vi "FrontPanel-4.50-backup.vi"() -> ()   [LabVIEW 2013]
doc: "This VI controls the blindpanel type GHS-2T-1T-700 for a CryoFree DR. Automatization control is embedded in the blindpanel. Keys can be manipulated from within this VI."
uses:
  Leiden to DSC/FP to DSC/Typedefs/FP-cluster.ctl
  1. Sources/Lib/Lib.llb/ErrCodeStatusLkup.vi
  1. Sources/Lib/Lib.llb/Pfeiffer Vacuum.lvlib
  1. Sources/Lib/Lib.llb/MView.lvlib
  1. Sources/Lib/Lib.llb/Busy PopUp.lvlib
panel:
  out "VIRef":T1 {"Array DataType" format="%.0x"; "WaveForm Type" format="%.0x"; "RefNum Type" format="%.0x"; "DataType" format="%.0x"}
  out "ControlNames":string[](array[string])
  in  "Toolbar":enum32{"Page 1", "Page 2"}(tab)
  in  "Load config":bool
  in  "Save config":bool
  in  "Start":bool
  in  "Stop":bool
  out "V":string
  out "PT2 Data":dbl[](array[numeric])
  in  "Restart PT on Error?":bool
  in  "Attempts":u16=6
  in  "Time delay":u16=60 format="%.0f s"
  out "Error Log":string[][](table)
  in  "Error panel":enum32{"Page 1"}(tab)
  out "PT2 error":errorcluster
  out "MG error":errorcluster
  out "PT1 error":errorcluster
  out "FP error":errorcluster
  out "PT1 Data":dbl[](array[numeric])
  in  "Main Panel":enum32{"Page 1", "Page 2"}(tab)
  out "PC":sgl
  out "P1":sgl format="%.1f"
  out "P2":sgl format="%.1f"
  out "P3":sgl format="%.1f"
  out "P4":sgl format="%.1f"
  out "P5":sgl format="%.1f"
  out "P6":sgl format="%.1f"
  out "P7":sgl format="%.1f"
  out "Flow":sgl format="%#_4f"
  out "P5 alarm":bool
  out "Pstill (P8)":dbl format="%.1e"
  in  "Main Panel":T2(tab)
  out "String 2":string
  out "String 4":string
  out "String":string
  out "String 3":string
  out "Mode":u16(ring) items=["AUTO MODE OFF", "START", "CONDENSING 3He", "CONDENSING 4He", "NORMAL CIRCULATION", "RECOVERY OF THE MIXTURE", "RECOVERY: BLOCKAGE OR OVERPRESSURE"]
  out "FLOW":sgl format="%#_3f"
  out "P5":sgl
  out "P4":sgl
  out "P3":sgl
  out "P1":sgl
  out "P2":sgl
  out "3He":sgl(slide) min=0 max=2 scale=0.0..2000.0 scale format="%.2f"
  out "4He":sgl(slide) min=0 max=2 scale=0.0..2000.0 scale format="%.2f"
  out "Panel ID":string
  in  "FP type":enum32{"OLD", "NEW"}(tab)
  in  "Buttons":T3
  out "LEDs":T4
  in  "Buttons 2":T3
  out "LEDs 2":T5
  out "PC":sgl
  in  "PT Start 2":bool
  in  "PT_stop 2":bool
  in  "PT2 Plots Select":T6
  out "PT2 Status":cluster{"Time":dbl[], "Value":dbl[]}[](graph)
  in  "PT_ResetValues 2":bool
  out "PT Error Code 2":i32 caption="PT Error Code"
  out "PT Error 2":string="NO ERROR" caption="PT Error"
  out "P High":cluster{dbl, dbl, dbl, dbl}(slide) scale=150.0..450.0
  out "P Low":cluster{dbl, dbl, dbl, dbl}(slide) scale=0.0..300.0
  out "P_avg 2":cluster{"Low":dbl, "High":dbl} caption="Average pressure"
  out "Helium":cluster{dbl, dbl, dbl, dbl}(slide) scale=0.0..95.0
  out "Water In":cluster{dbl, dbl, dbl, dbl}(slide) scale=0.0..35.0
  out "Water Out":cluster{dbl, dbl, dbl, dbl}(slide) scale=0.0..60.0
  out "PT Status":u16(ring) items=["Compressor OFF", "Compressor ON", ""]
  out "Motor":cluster{dbl, dbl}(slide) scale=0.0..30.0
  out "Oil":cluster{dbl, dbl, dbl, dbl}(slide) scale=0.0..60.0
  in  "PT1 Plots Select":T6
  out "PT1 Status 2":cluster{"Time":dbl[], "Value":dbl[]}[](graph)
  out "P Low":cluster{dbl, dbl, dbl, dbl}(slide) scale=0.0..300.0
  out "P High":cluster{dbl, dbl, dbl, dbl}(slide) scale=150.0..450.0
  out "P_avg":cluster{"Low":dbl, "High":dbl} caption="Average pressure"
  out "Motor":cluster{dbl, dbl}(slide) scale=0.0..30.0
  out "Oil":cluster{dbl, dbl, dbl, dbl}(slide) scale=0.0..60.0
  out "Helium":cluster{dbl, dbl, dbl, dbl}(slide) scale=0.0..95.0
  out "Water Out":cluster{dbl, dbl, dbl, dbl}(slide) scale=0.0..60.0
  out "Water In":cluster{dbl, dbl, dbl, dbl}(slide) scale=0.0..35.0
  out "PT Error Code":i32
  out "PT Error":string="NO ERROR"
  in  "PT_ResetValues":bool
  in  "PT Start":bool
  in  "PT_stop":bool
  out "PT Status":u16(ring) items=["Compressor OFF", "Compressor ON", ""]
  in  "MG Plots Select":T6
  in  "FP Plots Select":T6
  out "MaxiGauge":cluster{"Time":dbl[], "Value":dbl[]}[](graph)
  out "Front Panel":cluster{"Time":dbl[], "Value":dbl[]}[](graph)
  in  "Boolean 2":bool
  out "PT2 port":u16
  out "PT1 port":u16
  out "MG port":refnum<visa-resource-name>="COM4" caption="Port number"
  out "FP port":refnum<visa-resource-name>="COM3" caption="Port number"
  out "ForceSave":bool
  in  "Button":u8
  out "SetControl":T7
  in  "S2":enum32{"Page 1"}(tab)
  in  "Reset Error 2":bool
  in  "S1":enum32{"Page 1"}(tab)
  in  "Reset Error":bool
  out "Cur Path":path
  in  "Side Panel":enum32{"Main", "Settings", "Advanced"}(tab)=enum."Settings"
  out "Maxigauge ID":string caption="ID"
  out "Panel response":string
  out "Sensors Status":T8={"String 8"="OK", "String 9"="OK", "String 10"="OK", "String 11"="OK", "String 12"="OK", "String 13"="OK"}
  in  "ADC scaling":T9={"P1"=2500.0, "P2"=2500.0, "P3"=2500.0, "P4"=2500.0, "P5"=2500.0, "P6"=2500.0, "P7"=2500.0, "Flow meter"=682.0, "PC"=10000.0} caption="Front panel ADC scaling factors" {"Flow meter" format="%#.4f"}
  in  "REC Settings":T10={"P6 low"=20, "P6 high"=1000, "P7 low"=20}
  in  "NCP5B Settings":cluster{"P6 low":u16}={"P6 low"=20}
  in  "NCP5 Settings":T10={"P6 low"=20, "P6 high"=1000, "P7 low"=20}
  in  "S1&2 Settings":cluster{"Enum":enum16{"OFF", "ON"}}
  in  "P5 Settings":cluster{"P6 low":u16, "P6 high":u16}={"P6 low"=20, "P6 high"=1000}
  out "REC limits":T11={"P5 warn"=20, "P5 rec"=20, "P5 res"=20}
  out "NCP5B limits":cluster{"P5 NC4":u16}={"P5 NC4"=20}
  out "NCP5 limits":T12={"P5 NC1"=20, "P5 NC2"=20, "P5 NC3"=20}
  out "S1&2 limits":cluster{"S1&S2":enum16{"OFF", "ON"}}
  out "P5 limits":cluster{"P5 C1":u16, "P5 C2":u16}={"P5 C1"=20, "P5 C2"=20}
  in  "P6&7 Settings":T13={"P6 low"=20, "P6 high"=1600, "P7 low"=20, "P7 high"=1610}
  out "P6&7 limits":T13={"P6 low"=20, "P6 high"=20, "P7 low"=20, "P7 high"=20}
  in  "SET VALUES":bool
  out "MG pressures":T14 {"Channel 1" format="%-7.2e mbar"; "Channel 1" format="%-7.2e mbar"; "Channel 1" format="%-7.2e mbar"; "Channel 1" format="%-7.2e mbar"; "Channel 1" format="%-7.2e mbar"; "Channel 1" format="%-7.2e mbar"}
  out "Cluster":T15={"String 2"="\"\"", "String 3"="", "String 4"="", "String 5"="", "String 6"="", "String 7"=""}
  in  "Log Options":T16={"Plot data "=TRUE, "Every1"=1.0, "Save to log"=TRUE, "Every  2"=1.0, "AVS_Path 2"=path "C:/LC Data/Data", "AVS_FName"="logFP", "Filename suffix"="_%Y-%m-%d-%H-%M-%S", "NewFevery"=7, "Time Units"=enum."Days", "Date Format"="%Y-%m-%d %H:%M:%S", "Averages"=4} caption="Data Logging \nOptions" {"Every  2" format="%#_g min"; "Every1" format="%#_g min"}
  in  "Configuration":T17={"FP port number"="COM3", "MG port number"="COM4", "PT1 Enabled?"=FALSE, "MG  channel P8"=65535, "Stop auto recovery if still is empty"=FALSE, "PT1 port number"="COM2", "MG Enabled?"=TRUE, "PT1 Address"=16, "S1 Enabled?"=FALSE, "S1 port"="COM2", "S2 Enabled?"=FALSE, "S2 port"="COM2", "Device address S1"=1, "Device address S2"=2, "PT1 Bauds"=115200, "PT2 Enabled?"=FALSE, "PT2 port number"="COM2", "PT2 Address"=16, "PT2 Bauds"=115200, "FP baud rate"=9600} {"PT2 Address" min=16 max=126 step=1; "MG  channel P8" items=["Channel 1", "Channel 2", "Channel 3", "Channel 4", "Channel 5", "Channel 6"]; "PT1 Address" min=16 max=126 step=1}
  in  "Type":enum32{"Wet", "CF"}(radio)=enum."CF"
  in  "Panel Layout":enum32{"OLD", "NEW"}(ring)=enum."NEW"
  out "RAW ADC Values 2":dbl[](array[numeric]) caption="Converted ADC Values"
  in  "SendCMD":bool caption="Send"
  out "Response":string
  in  "Command":string
  out "SP reached? 2":bool
  in  "Cond1":bool
  in  "Delay Time":u32=30 caption="For a time delay of" format="%.0f min"
  in  "MG  channel":u16(ring)=65535 caption="MaxiGauge" items=["Channel 1", "Channel 2", "Channel 3", "Channel 4", "Channel 5", "Channel 6"]
  out "SP reached? 3":bool
  in  "P threshold":dbl=0.0005 caption="<" format="%#_2g mbar"
  in  "Cond2":bool
  out "SP reached?":bool
  out "Delay Timer":u32=10 caption="Timer" format="%<%M:%S>t"
  in  "EnableAutoCond":bool caption="Start"
  out "VI path":string
  out "RAW ADC Values":i32[](array[numeric])
  in  "Autoconf":bool caption="Autoconfigure"
  out "MG Data":dbl[](array[numeric]) format="%.3e"
  out "FP Data":sgl[](array[numeric]) format="%.2f"
  out "FP Status bits":u32[](array[numeric])
  out "Attempts Counter":u16
  # "Error log"
  # "Front panel status"
  # "MaxiGauge status"
  # "Pulse Tube 1 status"
  # "Pulse Tube 2 status"
  # "Leiden Cryogenics"
  # "to \nair"
  # "N.C."
  # "from\novc"
  # "from\nivc"
  # "from still"
  # "to 3He\nin-1"
  # "to 3He\nin-2"
  # "P8"
  # "AUX 1"
  # "BYPASS"
  # "MIXTURE\nCOMPRESSOR"
  # "M2"
  # "P6"
  # "M3"
  # "M1"
  # "AUX PORT-1"
  # "P7"
  # "TRAP"
  # "AUX TRAP"
  # "To \nAir"
  # "From\nIVC"
  # "From Still"
  # "To 3He\nin-1"
  # "To 3He\nin-2"
  # "To \nAir"
  # "N.C."
  # "from\novc"
  # "from\nivc"
  # "from still"
  # "to 3He\nin-1"
  # "to 3He\nin-2"
  # "Leiden Cryogenics"
  # "to \nair"
  # "N.C."
  # "from\novc"
  # "from\nivc"
  # "from still"
  # "to 3He\nin-1"
  # "to 3He\nin-2"
  # "P8"
  # "M2"
  # "P6"
  # "M3"
  # "TRAP"
  # "AUX TRAP"
  # "M1"
  # "AUX PORT-1"
  # "P7"
  # "AUX 1"
  # "To \nAir"
  # "From\nIVC"
  # "From Still"
  # "To 3He\nin-1"
  # "to 3He\nin-1"
  # "To 3He\nin-2"
  # "to \nair"
  # "N.C."
  # "from\novc"
  # "from\nivc"
  # "from still"
  # "to 3He\nin-2"
  # "Pulse Tube 1"
  # "Pulse Tube 2"
  # "Front Panel"
  # "MaxiGauge"
  # "Turbo2 (S2)"
  # "Turbo1 (S1)"
  # "MaxiGauge"
  # "#"
  # "NAME"
  # "PRESSURE"
  # "STATUS"
  # "1"
  # "2"
  # "3"
  # "4"
  # "5"
  # "6"
  # "Automatic mode pressure limits"
  # "Warning: These values influence the operation of the GHS in automatic mode. Please refer to the operation manual and consult with Leiden Cryogenics before changing them."
  # "NAME"
  # "FW"
  # "NEW"
  # "DESCRIPTION"
  # "Stop condensing 4He"
  # "Stop recovering 4He"
  # "Stop condensing 3He"
  # "Stop recovering 3He"
  # "Condensing->open 12"
  # "Condensing->close 9/12"
  # "Condensing->run S1&S2"
  # "NC->open second line"
  # "NC->start MC"
  # "NC->open aux. trap"
  # "NC->stop MC, close 7"
  # "All->P5 alarm"
  # "All->switch to recovery"
  # "All->reset"
  # "Front panel ADC scaling factors"
  # "Data Logging and Plotting"
  # "Front Panel"
  # "MaxiGauge"
  # "Pulse Tube 1"
  # "Pulse Tube 2"
  # "Turbo 1 (S1) (Pfeiffer HiPACE only)"
  # "Turbo2 (S2) (Pfeiffer HiPACE only)"
  # "Automatic condensing"
  # "Start condensing when"
  # "and wait"
  # "Send command to Front Panel"
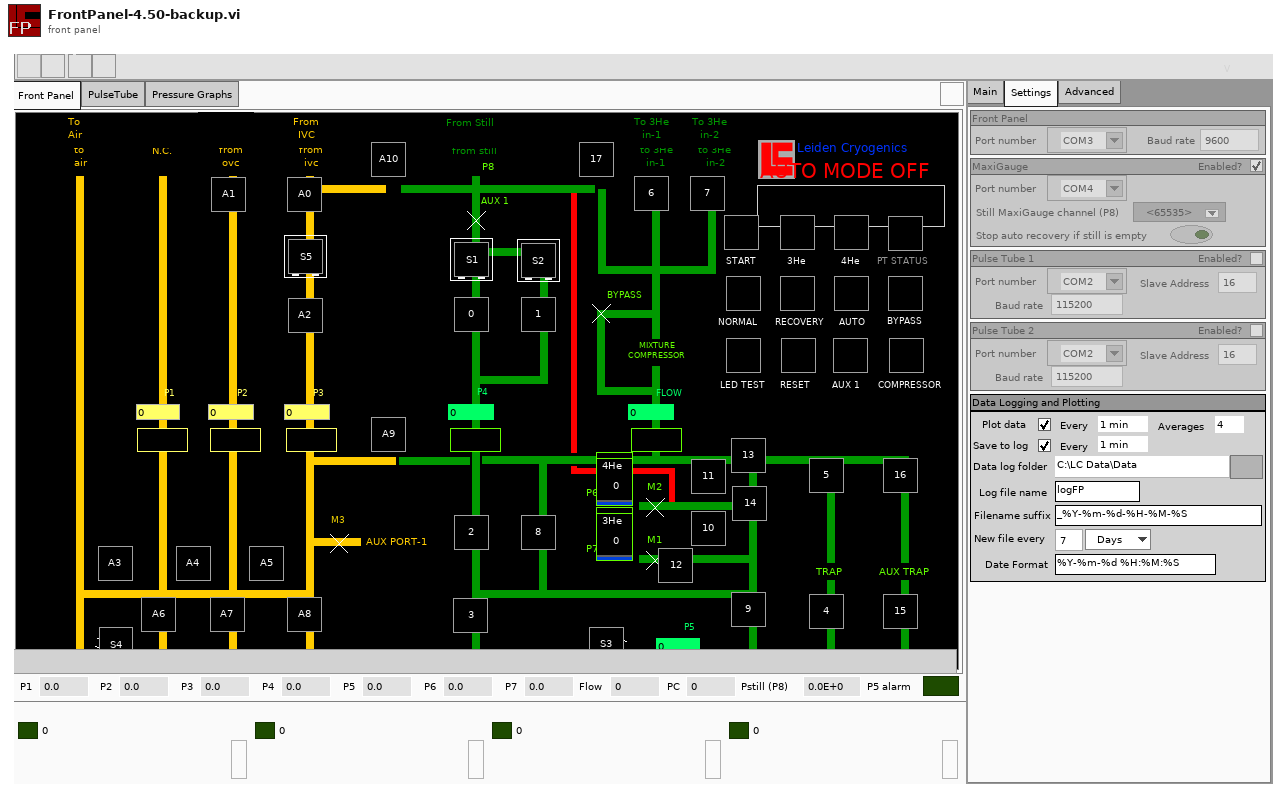
[diagram p1: front panel]
types:
  T1 = cluster{"Control Ref ID":refnum<vi>[], "Full Name":string[], "ClassID":enum16{"<Null>", "1", "2", "Generic", "Decoration", "Text", "Control", "ColorBox", "Boolean", "RefNum", "Variant", "Path", "ListBox", "Table", "Array", "Picture", "ActiveXContainer", "Numeric", "Digital", "NamedNumeric", "ColorRamp", "Slide", "GraphOrChart", "WaveformChart", "WaveformGraph", "IntensityChart", "IntensityGraph", "String", "IOName", "ComboBox", "Cluster", "Panel", "Knob", "NumWithScale", "Ring", "Enum", "GObject", "Plot", "Cursor", "NumericText", "Scale", "ColorScale", "GraphScale", "ColorGraphScale", "TypedRefNum", "OldKnobScale", "MCListbox", "MeasureData", "BVTag", "DAQName", "VISAName", "IVIName", "SlideScale", "TabControl", "Page", "TabArrayTabControl", "ConPane", "57", "58", "59", "60", "61", "62", "63", "64", "SubPanel", "TreeControl", "67", "68", "69", "70", "71", "72", "73", "74", "75", "SplitterBar"}[], "Short Name":string[], "DataType":enum8{"<Null>", "I8", "I16", "I32", "I64", "U8", "U16", "U32", "U64", "SGL", "DBL", "EXT", "CSG", "CDB", "CXT", "0x0F", "0x10", "0x11", "0x12", "0x13", "0x14", "Enum U8", "Enum U16", "Enum U32", "Enum U64", "SGL PQ", "DBL PQ", "EXT PQ", "CSG PQ", "CDB PQ", "CXT PQ", "0x1F", "0x20", "Boolean", "0x22", "0x23", "0x24", "0x25", "0x26", "0x27", "0x28", "0x29", "0x2A", "0x2B", "0x2C", "0x2D", "0x2E", "0x2F", "String", "0x31", "Path", "Pict", "0x34", "0x35", "0x36", "DAQ", "0x38", "0x39", "0x3A", "0x3B", "0x3C", "0x3D", "0x3E", "0x3F", "Array", "0x41", "0x42", "0x43", "0x44", "0x45", "0x46", "0x47", "0x48", "0x49", "0x4A", "0x4B", "0x4C", "0x4D", "0x4E", "0x4F", "Cluster", "0x51", "0x52", "Variant", "Waveform", "0x55", "0x56", "0x57", "0x58", "0x59", "0x5A", "0x5B", "0x5C", "0x5D", "0x5E", "0x5F", "0x60", "0x61", "0x62", "0x63", "0x64", "0x65", "0x66", "0x67", "0x68", "0x69", "0x6A", "0x6B", "0x6C", "0x6D", "0x6E", "0x6F", "Refnum"}[], "RefNum Type":enum8{"Generic", "Datalog File Refnum", "Byte Stream File Refnum", "Device Refnum", "Occurence Refnum", "TCP Connection Refnum", "VISA Refnum (Obsolete)", "Automation Renum", "VI Server Refnum", "Menu Refnum", "IVI Refnum (Obsolete)", "IMAQ Session", "0x0C", "Datasocket Refnum", "VISA Resource", "IVI Logical Name", "UDP Connection Refnum", "Notifier Refnum", "Queue Refnum", "IrDA Refnum", "Hardware Plugin Refnum", "Hardware Plugin Tag Refnum", "DAQmx Refnum", "Event Registration Refnum", ".NET Refnum", "User Event Refnum", "0x1A", "Event Callback", "0x1C", "0x1D", "Only Used Internal to LabVIEW", "Bluetooth", "Data Value References", "RT FIFO", "TDM Streaming"}[], "WaveForm Type":enum8{"<Not a Waveform Type>", "0x01", "Analog 16-bit signed", "Analog Double-Precision", "0x04", "Analog Single Precision", "Timestamp", "Digital Data", "Digital Waveform", "Dynamic Data", "Analog Extended-Precision", "Analog 8-bit unsigned", "Analog 16-bit unsigned", "Analog 32-bit unsigned", "Analog 8-bit signed", "Analog 32-bit signed", "Analog Complex Single-Precision", "Analog Complex Double-Precision", "Analog Complex Extended Precision", "Analog 64-bit signed", "Analog 64-bit unsigned"}[], "Parent":i32[], "Array DataType":enum8{"<Null>", "I8", "I16", "I32", "I64", "U8", "U16", "U32", "U64", "SGL", "DBL", "EXT", "CSG", "CDB", "CXT", "0x0F", "0x10", "0x11", "0x12", "0x13", "0x14", "Enum U8", "Enum U16", "Enum U32", "Enum U64", "SGL PQ", "DBL PQ", "EXT PQ", "CSG PQ", "CDB PQ", "CXT PQ", "0x1F", "0x20", "Boolean", "0x22", "0x23", "0x24", "0x25", "0x26", "0x27", "0x28", "0x29", "0x2A", "0x2B", "0x2C", "0x2D", "0x2E", "0x2F", "String", "0x31", "Path", "Pict", "0x34", "0x35", "0x36", "DAQ", "0x38", "0x39", "0x3A", "0x3B", "0x3C", "0x3D", "0x3E", "0x3F", "Array", "0x41", "0x42", "0x43", "0x44", "0x45", "0x46", "0x47", "0x48", "0x49", "0x4A", "0x4B", "0x4C", "0x4D", "0x4E", "0x4F", "Cluster", "0x51", "0x52", "Variant", "Waveform", "0x55", "0x56", "0x57", "0x58", "0x59", "0x5A", "0x5B", "0x5C", "0x5D", "0x5E", "0x5F", "0x60", "0x61", "0x62", "0x63", "0x64", "0x65", "0x66", "0x67", "0x68", "0x69", "0x6A", "0x6B", "0x6C", "0x6D", "0x6E", "0x6F", "Refnum"}[], "Owning VI":refnum<vi>[], "Active?":bool[]}
  T2 = enum32{"Front Panel", "PulseTube", "Pressure Graphs"}
  T3 = cluster{"baux2":bool, "bBypass":bool, "b15":bool, "b16":bool, "NC 0":bool, "baux1":bool, "b4":bool, "NC 1":bool, "b5":bool, "breset":bool, "NC 2":bool, "b9":bool, "b14":bool, "NC 3":bool, "b13":bool, "bledtest":bool, "NC 4":bool, "b12":bool, "b10":bool, "NC 5":bool, "b11":bool, "bA0":bool, "NC 9":bool, "b7":bool, "bS3":bool, "NC 12":bool, "b6":bool, "b17":bool, "NC 13":bool, "b8":bool, "b1":bool, "NC 14":bool, "bS2":bool, "b3":bool, "NC 15":bool, "b2":bool, "b0":bool, "NC 16":bool, "bS1":bool, "bA9":bool, "NC 17":bool, "bA8":bool, "bA2":bool, "NC 6":bool, "bs5":bool, "bA10":bool, "NC 7":bool, "bstart":bool, "bA5":bool, "NC 8":bool, "bA7":bool, "bA1":bool, "NC 10":bool, "bauto":bool, "bA4":bool, "NC 11":bool, "bA6":bool, "bS4":bool, "NC 18":bool, "bA3":bool, "b3he":bool, "b4he":bool, "bnorm":bool, "brecov":bool}
  T4 = cluster{"COMPR/AUX 2":bool, "BYPASS":bool, "15":bool, "16":bool, "NC 0":bool, "AUX 1":bool, "4":bool, "NC 1":bool, "5":bool, "RESET":bool, "NC 2":bool, "9":bool, "14":bool, "NC 3":bool, "13":bool, "LED TEST":bool, "NC 4":bool, "12":bool, "10":bool, "NC 5":bool, "11":bool, "A0":bool, "NC 12":bool, "7":bool, "S3":bool, "NC 13":bool, "6":bool, "17":bool, "NC 14":bool, "8":bool, "1":bool, "NC 15":bool, "S2":bool, "3":bool, "NC 16":bool, "2":bool, "0":bool, "NC 17":bool, "S1":bool, "A9":bool, "NC 6":bool, "A8":bool, "A2":bool, "NC 7":bool, "S5":bool, "A10":bool, "NC 8":bool, "START":bool, "A5":bool, "NC 9":bool, "A7":bool, "A1":bool, "NC 10":bool, "AUTO":bool, "A4":bool, "NC 11":bool, "A6":bool, "S4":bool, "NC 18":bool, "A3":bool, "3He":bool, "4He":bool, "NORMAL":bool, "RECOVERY":bool, "PT STATUS":bool}
  T5 = cluster{"COMPR/AUX 2":bool, "BYPASS":bool, "15":bool, "16":bool, "AUX 1":bool, "AUX 1":bool, "4":bool, "AUX 2":bool, "5":bool, "RESET":bool, "AUX 3":bool, "9":bool, "14":bool, "NC 3":bool, "13":bool, "LED TEST":bool, "NC 4":bool, "12":bool, "10":bool, "NC 5":bool, "11":bool, "A0":bool, "NC 12":bool, "7":bool, "S3":bool, "NC 13":bool, "6":bool, "17":bool, "NC 14":bool, "8":bool, "1":bool, "NC 15":bool, "S2":bool, "3":bool, "NC 16":bool, "2":bool, "0":bool, "NC 17":bool, "S1":bool, "A9":bool, "NC 6":bool, "A8":bool, "A2":bool, "NC 7":bool, "S5":bool, "A10":bool, "NC 8":bool, "START":bool, "A5":bool, "NC 9":bool, "A7":bool, "A1":bool, "NC 10":bool, "AUTO":bool, "A4":bool, "NC 11":bool, "A6":bool, "S4":bool, "NC 18":bool, "A3":bool, "3He":bool, "4He":bool, "NORMAL":bool, "RECOVERY":bool, "PT STATUS":bool}
  T6 = cluster{"Boolean":bool, "Boolean 2":bool, "Boolean 3":bool, "Boolean 4":bool, "Boolean 5":bool, "Boolean 6":bool, "Boolean 7":bool, "Boolean 8":bool}
  T7 = cluster{"Name":string, "Scalar":string, "Array":string[][]}
  T8 = cluster{"String 8":string, "String 9":string, "String 10":string, "String 11":string, "String 12":string, "String 13":string}
  T9 = cluster{"P1":dbl, "P2":dbl, "P3":dbl, "P4":dbl, "P5":dbl, "P6":dbl, "P7":dbl, "Flow meter":dbl, "PC":dbl}
  T10 = cluster{"P6 low":u16, "P6 high":u16, "P7 low":u16}
  T11 = cluster{"P5 warn":u16, "P5 rec":u16, "P5 res":u16}
  T12 = cluster{"P5 NC1":u16, "P5 NC2":u16, "P5 NC3":u16}
  T13 = cluster{"P6 low":u16, "P6 high":u16, "P7 low":u16, "P7 high":u16}
  T14 = cluster{"Channel 1":dbl, "Channel 1":dbl, "Channel 1":dbl, "Channel 1":dbl, "Channel 1":dbl, "Channel 1":dbl}
  T15 = cluster{"String 2":string, "String 3":string, "String 4":string, "String 5":string, "String 6":string, "String 7":string}
  T16 = cluster{"Plot data ":bool, "Every1":dbl, "Save to log":bool, "Every  2":dbl, "AVS_Path 2":path, "AVS_FName":string, "Filename suffix":string, "NewFevery":u32, "Time Units":enum16{"Minutes", "Hours", "Days"}, "Date Format":string, "Averages":i32}
  T17 = cluster{"FP port number":refnum<visa-resource-name>, "MG port number":refnum<visa-resource-name>, "PT1 Enabled?":bool, "MG  channel P8":u16, "Stop auto recovery if still is empty":bool, "PT1 port number":refnum<visa-resource-name>, "MG Enabled?":bool, "PT1 Address":u8, "S1 Enabled?":bool, "S1 port":refnum<visa-resource-name>, "S2 Enabled?":bool, "S2 port":refnum<visa-resource-name>, "Device address S1":u8, "Device address S2":u8, "PT1 Bauds":u32, "PT2 Enabled?":bool, "PT2 port number":refnum<visa-resource-name>, "PT2 Address":u8, "PT2 Bauds":u32, "FP baud rate":u32}
  T18 = cluster{"error":bool, "code":i32, "source":string}
  T19 = cluster{"Dict. Var":u16, "Description":string, "Values":i32[]}[]
  T20 = cluster{"[3]":dbl, "[3]":dbl, "[3]":dbl, "Values[3] 2":dbl}
  T21 = cluster{"[1]":dbl, "[1]":dbl, "[1]":dbl, "Values[1] 2":dbl}
  T22 = cluster{"Values[0]":dbl, "Values[0]":dbl, "Values[0]":dbl, "Values[0] 2":dbl}
  T23 = cluster{"error":bool, "code":i32, "error source":string}
  T24 = cluster{"sensor status info[0]":string, "sensor status info[1]":string, "sensor status info[2]":string, "sensor status info[3]":string, "sensor status info[4]":string, "sensor status info[5]":string}
  T25 = cluster{"Filterred[0]":dbl, "Filterred[1]":dbl, "Filterred[2]":dbl, "Filterred[3]":dbl, "Filterred[4]":dbl, "Filterred[5]":dbl}
  T26 = typedef "FP-cluster.ctl" = cluster{"FP Data":sgl[], "MG Data":dbl[], "PT Data":dbl[], "FP Status Bits":u32[], "Mode":u16}
  T27 = cluster{"FP Data[0]":sgl, "FP Data[1]":sgl, "FP Data[2]":sgl, "FP Data[3]":sgl, "FP Data[4]":sgl, "FP Data[5]":sgl, "FP Data[6]":sgl, "FP Data[7]":sgl, "FP Data[8]":sgl}
  T28 = enum32{"Page Enabled", "Page Disabled", "Page Disabled & Grayed"}
  T29 = enum32{"invalid app kind", "Development System", "Run Time System", "Student Edition", "Embedded LabVIEW", "Evaluation", "Custom"}
  T30 = cluster{"array of 4 x 16 bit unsigned[0]":u16, "array of 4 x 16 bit unsigned[1]":u16, "array of 4 x 16 bit unsigned[2]":u16, "array of 4 x 16 bit unsigned[3]":u16}
  T31 = cluster{"array of 2 x 16 bit unsigned[0]":u16, "array of 2 x 16 bit unsigned[1]":u16}
  T32 = cluster{"array of 3 x 16 bit unsigned[0]":u16, "array of 3 x 16 bit unsigned[1]":u16, "array of 3 x 16 bit unsigned[2]":u16}
  T33 = cluster{"Array[0]":string, "Array[1]":string, "Array[2]":string, "Array[3]":string, "Array[4]":string, "Array[5]":string}
  T34 = typedef "LVRectTypeDef.ctl" = cluster{"Left":i16, "Top":i16, "Right":i16, "Bottom":i16}
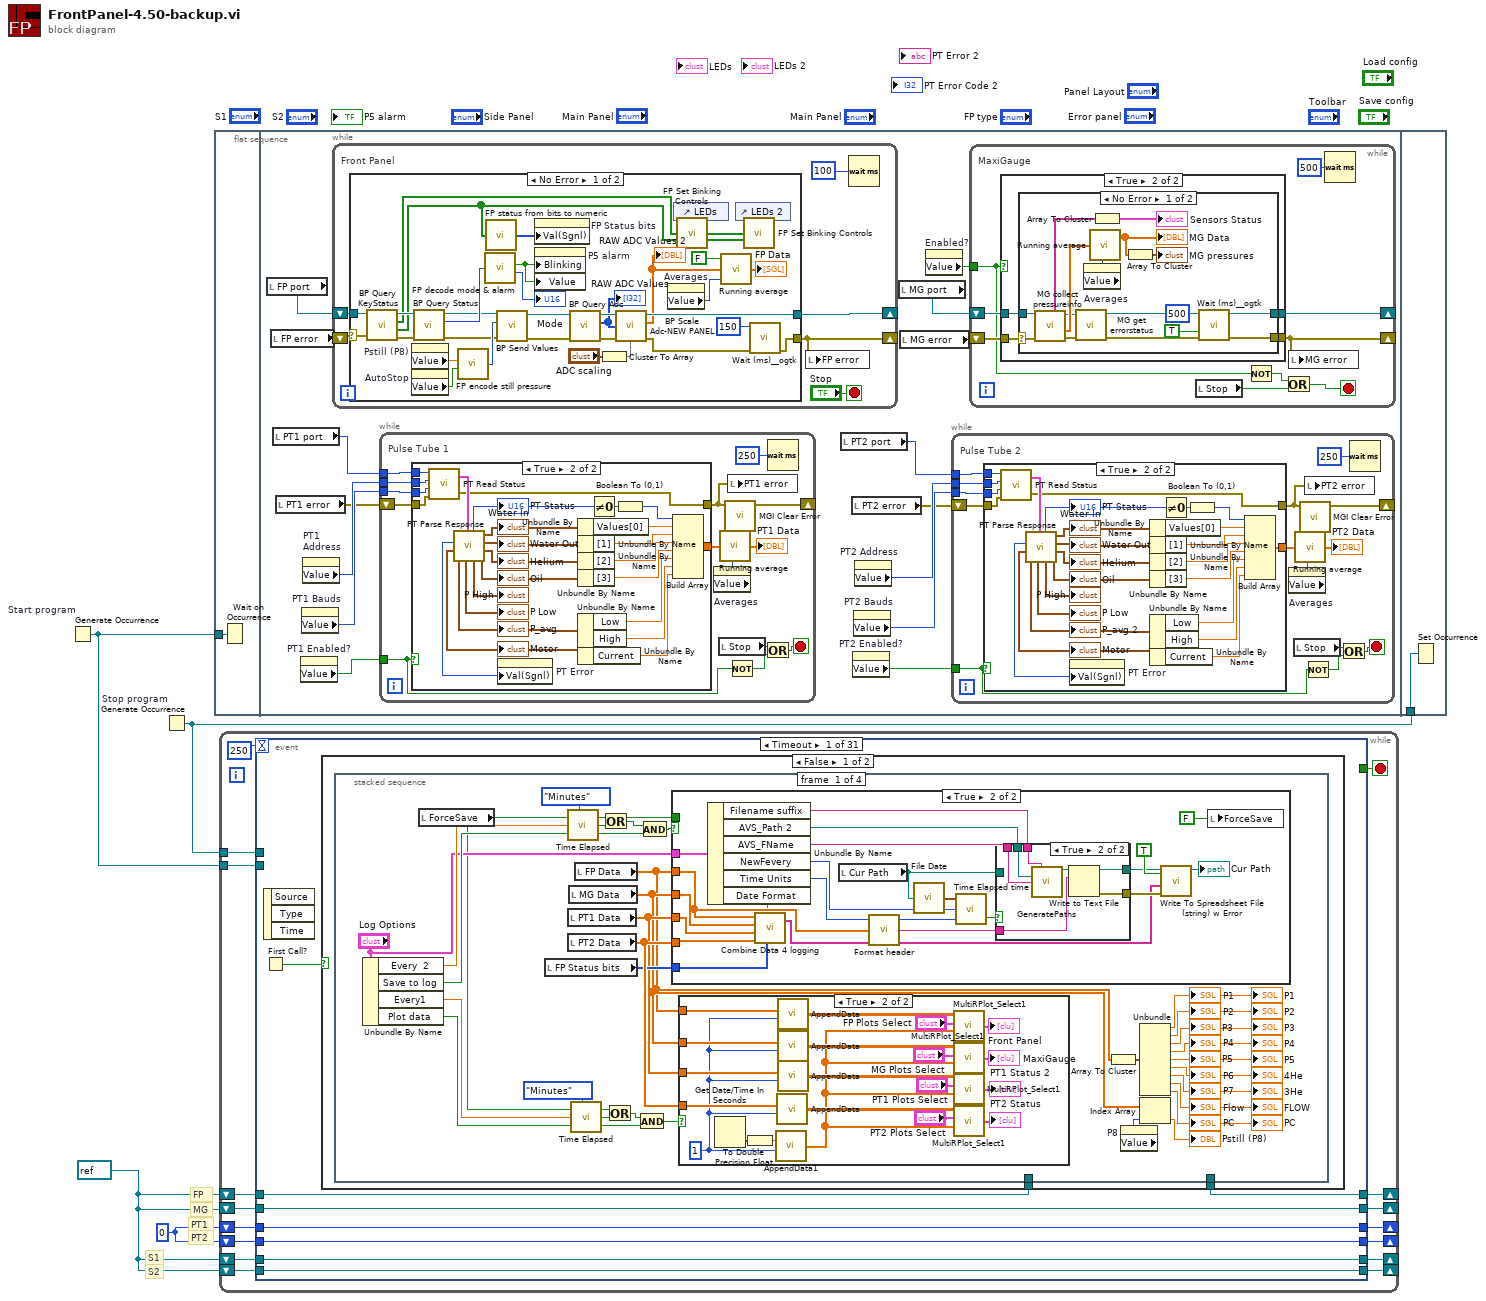
[diagram p0: block diagram]
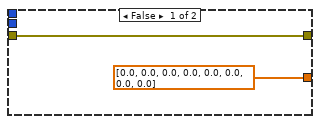
[diagram p2: hidden frame]
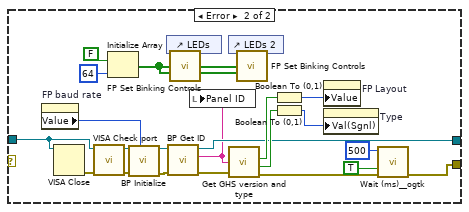
[diagram p3: hidden frame]
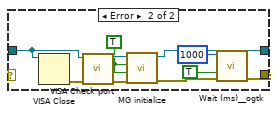
[diagram p5: hidden frame]
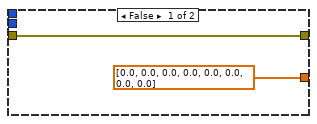
[diagram p6: hidden frame]
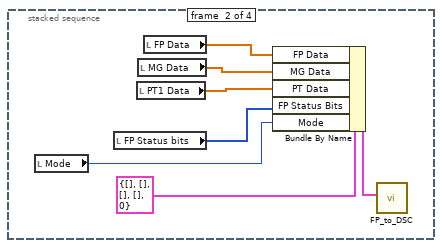
[diagram p10: hidden frame]
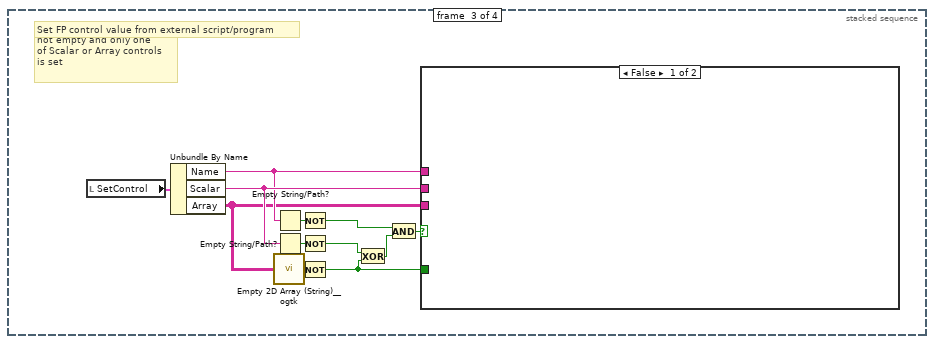
[diagram p11: hidden frame]
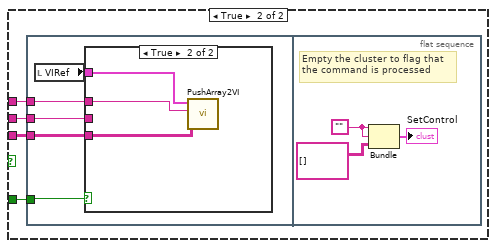
[diagram p12: hidden frame]
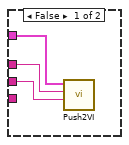
[diagram p13: hidden frame]
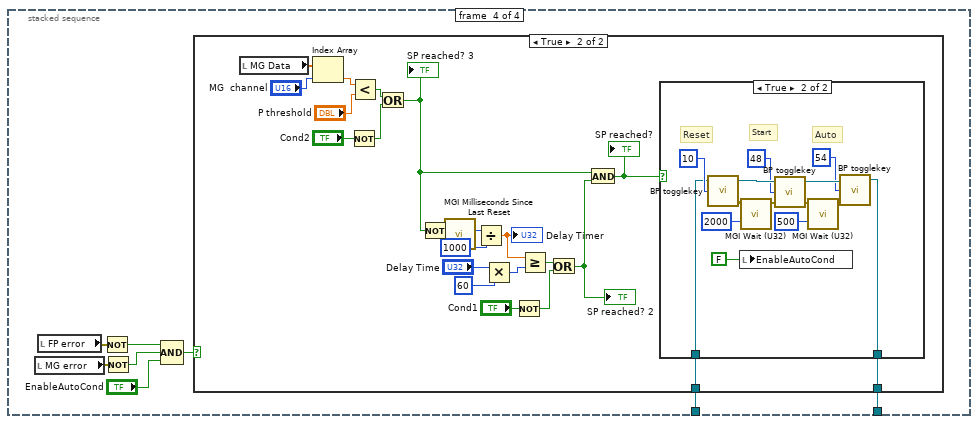
[diagram p14: hidden frame]
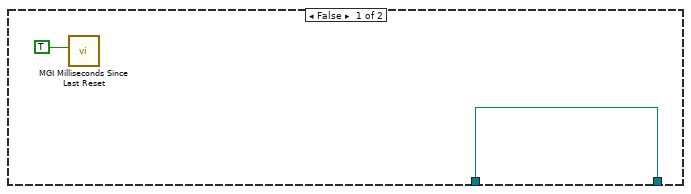
[diagram p15: hidden frame]
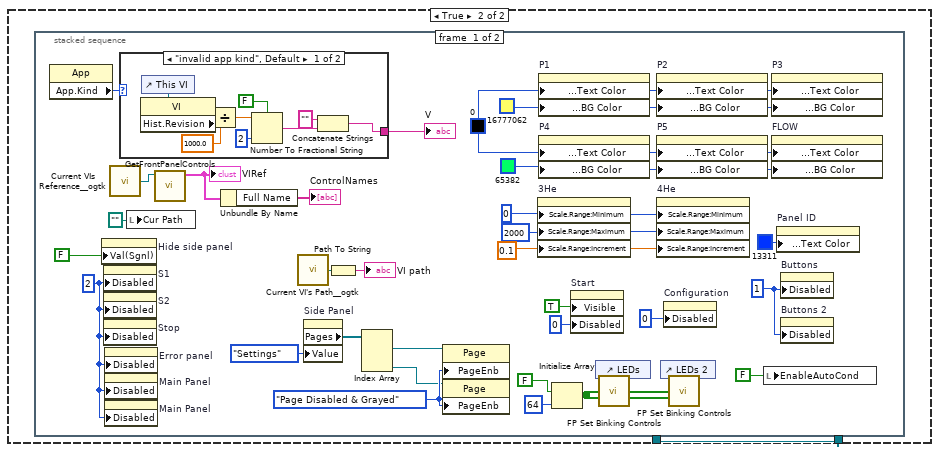
[diagram p17: hidden frame]
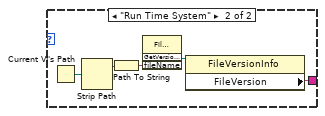
[diagram p18: hidden frame]
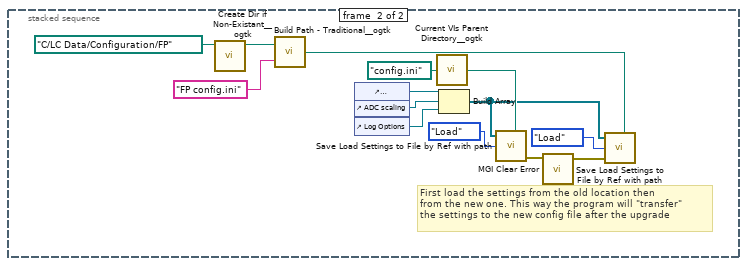
[diagram p19: hidden frame]
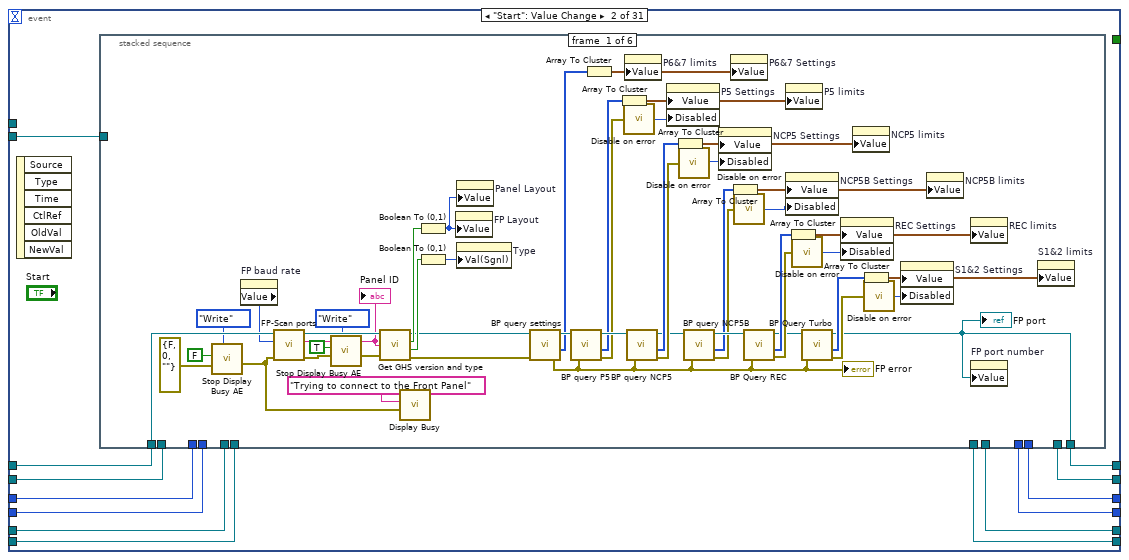
[diagram p20: hidden frame]
diagram:
  w1 = u8 0 ("x+1")
  w2 = refnum<visa-resource-name> refnum ("PT port")
  # "S2"
  # "S1"
  # "MG"
  # "PT1"
  # "PT2"
  # "FP"
  n1 = Generate Occurrence "Start program"() -> (w4:refnum<k4>)
  n2 = Generate Occurrence "Stop program"() -> (w3:refnum<k4>)
  n3 = flat-sequence {
    tunnel: w4 -> [w5]
    tunnel: w3 -> [w204]
    frame #0 {
      n4 = Wait on Occurrence(2:w5) -> ()  [unwired: 2 in, 1 out]
    }
    frame #1 {
      n5 = local read "FP port"() -> (w11:refnum<visa-resource-name>)
      n6 = local read "FP error"() -> (w16:errorcluster)
      n7 = local read "PT1 port"() -> (w7:u16)
      n8 = local read "PT1 error"() -> (w8:errorcluster)
      n9 = property on="PT1 Enabled?" class="Bool (strict)"() -> ("Value"=w19:bool)  [unwired: 2 in, 2 out]
      n10 = property on="PT1 Bauds" class="DigNum (strict)"() -> ("Value"=w17:u32)  [unwired: 2 in, 2 out]
      n11 = property on="PT1 \nAddress" class="DigNum (strict)"() -> ("Value"=w20:u8)  [unwired: 2 in, 2 out]
      n12 = while {
        shift-right: [w66] -> _
        shift-left: w16 -> [w67]
        shift-right: [w64] -> _
        shift-left: w11 -> [w65]
        stop <- "Stop" stop-if-true
        # "Front Panel"
        n13 = case shown="No Error" w67 {
          selector: w67 -> [w97 _]
          tunnel: [w78 w111] -> w64
          tunnel: [w76 w109] -> w66
          tunnel: w65 -> [w98 w112]
          frame No Error {
            n14 = call "BP Query KeyStatus.vi"("error in"=w97, "FrontPanel port"=w98) -> ("error out"=w86:T18, "Button states"=w69:bool[], "Blinking States"=w70:bool[], "FrontPanel port"=w87:refnum<visa-resource-name>)  [unwired: 2 in]
            n15 = property on="Pstill (P8)" class="DigNum (strict)"() -> ("Value"=w88:dbl)  [unwired: 2 in, 2 out]
            n16 = property on="AutoStop" class="Bool (strict)"() -> ("Value"=w89:bool)  [unwired: 2 in, 2 out]
            n17 = call "BP Query Status.vi"("error in"=w86, "FrontPanel port"=w87) -> ("error out"=w91:T18, "status word (32 bit unsigned)"=w94:u32, "FrontPanel port"=w92:refnum<visa-resource-name>)  [unwired: 3 in]
            n18 = call "FP encode still pressure.vi"("Value 2"=w89, "Value"=w88) -> ("Numeric"=w93:u16)  [unwired: 4 in]
            n19 = call "FP decode mode & alarm.vi"("status word (32 bit unsigned)"=w94) -> ("Boolean"=w90:bool, "Numeric"=→"Mode":u32)  [unwired: 4 in]
            n20 = call "FP status from bits to numeric.vi"("FP Status bits"=w69) -> ("FP status number"=w96:u32[])  [unwired: 4 in]
            n21 = call "BP Send Values.vi"("error in"=w91, "value to send"=w93, "FrontPanel port"=w92) -> ("error out"=w80:T18, "FrontPanel port"=w81:refnum<visa-resource-name>)  [unwired: 3 in]
            n22 = property on="FP Status bits" class="Arr (strict)"("Val(Sgnl)"=w96) -> ()  [unwired: 2 in, 2 out]
            n23 = property on="P5 alarm" class="Bool (strict)"("Blinking"=w90, "Value"=w90) -> ()  [unwired: 2 in, 2 out]
            n24 = call "BP Query Adc.vi"("error in"=w80, "FrontPanel port"=w81) -> ("error out"=w77:T18, "array of 8(9) x 16 bit signed"=w72:i32[], "FrontPanel port"=w78:refnum<visa-resource-name>)  [unwired: 3 in]
            "RAW ADC Values" <- w72
            n25 = Cluster To Array(cluster="ADC scaling") -> (array=w79:dbl[])
            n26 = call "BP Scale Adc-NEW PANEL.vi"("input array scaling factors,8(9) x 16 bit uint"=w79, "input array 8(9) x 16bit uint"=w72) -> ("output array 8(9) x single prec. incl flow"=w71:sgl[])  [unwired: 4 in, 1 out]
            "RAW ADC Values 2" <- w71
            n27 = property on="Averages" class="DigNum (strict)"() -> ("Value"=w85:i32)  [unwired: 2 in, 2 out]
            n28 = control-ref of="LEDs"() -> (w74:refnum<vi>)
            n29 = call "FP Set Binking Controls.vi"("Cluster in"=w74, "Array of blinking states"=w70, "Array of relais states"=w69) -> ()  [unwired: 13 in]
            n30 = call "Running average.vi"("Window Size"=w85, "New values"=w71, "Filter Zeroes? (T)"=FALSE) -> ("Filterred"=→"FP Data":dbl[])  [unwired: 1 in]
            n31 = control-ref of="LEDs 2"() -> (w73:refnum<vi>)
            n32 = call "FP Set Binking Controls.vi"("Cluster in"=w73, "Array of blinking states"=w70, "Array of relais states"=w69) -> ()  [unwired: 13 in]
            n33 = call "Wait (ms)__ogtk.vi"("error in (no error)"=w77, "milliseconds to wait"=u32 150) -> ("error out"=w76:errorcluster)  [unwired: 8 in, 1 out]
          }
          frame Error {
            n34 = property on="FP baud rate" class="DigNum (strict)"() -> ("Value"=w104:u32)  [unwired: 2 in, 2 out]
            n35 = VISA Close(VISA resource name=w112) -> (error out=w121:errorcluster)  [unwired: 1 in]
            n36 = call "VISA Check port.vi"("error in (no error)"=w121, "VISA Resource Name in"=w112) -> ("error out"=w120:errorcluster, "VISA Resource Name out"=w119:refnum<visa-resource-name>)  [unwired: 8 in]
            n37 = Initialize Array(FALSE, 64 ("dimension size")) -> (w99:bool[])
            n38 = call "BP Initialize.vi"("FP baud rate"=w104, "error in (no error)"=w120, "FrontPanel port"=w119) -> ("error out"=w118:errorcluster, "FrontPanel port"=w117:refnum<visa-resource-name>)  [unwired: 4 in]
            n39 = control-ref of="LEDs"() -> (w101:refnum<vi>)
            n40 = call "BP Get ID.vi"("error in (no error)"=w118, "FrontPanel port"=w117) -> ("error out"=w106:errorcluster, "Device ID string"=w110:string, "FrontPanel port"=w111:refnum<visa-resource-name>)  [unwired: 6 in, 1 out]
            n41 = call "FP Set Binking Controls.vi"("Cluster in"=w101, "Array of blinking states"=w99, "Array of relais states"=w99) -> ()  [unwired: 13 in]
            n42 = local write "Panel ID"(w110) -> ()
            n43 = control-ref of="LEDs 2"() -> (w100:refnum<vi>)
            n44 = call "Get GHS version and type.vi"("ID string"=w110, "error in (no error)"=w106) -> ("Panel Version"=w113:bool, "System Type"=w115:bool, "error out"=w105:errorcluster)  [unwired: 4 in]
            n45 = call "FP Set Binking Controls.vi"("Cluster in"=w100, "Array of blinking states"=w99, "Array of relais states"=w99) -> ()  [unwired: 13 in]
            n46 = Boolean To (0,1)(Boolean=w113) -> (0, 1=w114:i16)
            n47 = Boolean To (0,1)(Boolean=w115) -> (0, 1=w116:i16)
            n48 = property on="FP Layout" class="TabCtl (strict)"("Value"=w114) -> ()  [unwired: 2 in, 2 out]
            n49 = property on="Type" class="RadioBtnsControl (strict)"("Val(Sgnl)"=w116) -> ()  [unwired: 2 in, 2 out]
            n50 = call "Wait (ms)__ogtk.vi"("error in (no error)"=w105, "Wait on Error (FALSE)"=TRUE, "milliseconds to wait"=u32 500) -> ("error out"=w109:errorcluster)  [unwired: 7 in, 1 out]
          }
        }
        n51 = local write "FP error"(w66) -> ()
        n52 = Wait (ms)(milliseconds to wait=u32 100) -> ()  [unwired: 1 out]
      }
      n53 = while {
        tunnel: w7 -> [w174]
        tunnel: w20 -> [w173]
        tunnel: w19 -> [w164]
        tunnel: w17 -> [w170]
        shift-right: [w163] -> _
        shift-left: w8 -> [w169]
        stop <- w167 stop-if-true
        # "Pulse Tube 1"
        n54 = case shown="True" w164 {
          tunnel: [dbl[] [0.0, 0.0, 0.0, 0.0, 0.0, 0.0, 0.0, 0.0] w191] -> w175
          tunnel: w174 -> [_ w190]
          tunnel: w169 -> [w176 w189]
          tunnel: w173 -> [_ w188]
          tunnel: w170 -> [_ w183]
          tunnel: [w176 w182] -> w162
          frame False {
          }
          frame True {
            n55 = call "PT Read Status.vi"("error in (no error)"=w189, "Baud"=w183, "Slave Address"=w188, "Com Port #"=w190) -> ("error out"=w182:errorcluster, "Response"=w192:T19)
            n56 = call "PT Parse Response.vi"("Response"=w192) -> ("Oil temp"=w197:T20, "He temp"=w196:cluster{"[2]":dbl, "[2]":dbl, "[2]":dbl, dbl}, "Out water temp"=w195:T21, "In water temp"=w194:T22, "P_high"=→"P High":cluster{"[0]":dbl, "[0]":dbl, "[0]":dbl, dbl}, "Numeric"=w201:i32, "P_low"=→"P Low":cluster{"[1]":dbl, "[1]":dbl, "[1]":dbl, dbl}, "Average pressure"=w187:cluster{"Low":dbl, "High":dbl}, "Current"=w181:cluster{"Current":dbl, "Threshold":dbl}, "PT Error"=w193:i32)  [unwired: 1 in]
            "Oil" <- w197
            "Motor" <- w181
            "PT Status" <- w201
            "Water Out" <- w195
            "Water In" <- w194
            "Helium" <- w196
            "P_avg" <- w187
            n57 = property on="PT Error" class="DigNum (strict)"("Val(Sgnl)"=w193) -> ()  [unwired: 2 in, 2 out]
            n58 = Unbundle By Name(w194) -> ("Values[0]"=w184:dbl)
            n59 = Unbundle By Name(w195) -> ("[1]"=w200:dbl)
            n60 = Unbundle By Name(w196) -> ("[2]"=w199:dbl)
            n61 = Unbundle By Name(w197) -> ("[3]"=w198:dbl)
            n62 = Unbundle By Name(w187) -> ("Low"=w186:dbl, "High"=w185:dbl)
            n63 = Unbundle By Name(w181) -> ("Current"=w180:dbl)
            n64 = Not Equal To 0?(x=w201) -> (x != 0?=w202:bool)
            n65 = Boolean To (0,1)(Boolean=w202) -> (0, 1=w203:i16)
            n66 = Build Array(w203, w184, w200, w199, w198, w186, w185, w180) -> (w191:dbl[])
          }
        }
        n67 = property on="Averages" class="DigNum (strict)"() -> ("Value"=w172:i32)  [unwired: 2 in, 2 out]
        n68 = local read "Stop"() -> (w166:bool)
        n69 = call "Running average.vi"("Window Size"=w172, "New values"=w175) -> ("Filterred"=→"PT1 Data":dbl[])  [unwired: 2 in]
        n70 = call "MGI Clear Error.vi"("Error In"=w162) -> ("Error Out"=w163:errorcluster)  [unwired: 6 in]
        n71 = Not(x=w164) -> (.not. x?=w165:bool)
        n72 = local write "PT1 error"(w162) -> ()
        n73 = Or(x=w166, y=w165) -> (x .or. y?=w167:bool)
        n74 = Wait (ms)(milliseconds to wait=u32 250) -> ()  [unwired: 1 out]
      }
      n75 = local read "PT2 port"() -> (w6:u16)
      n76 = local read "PT2 error"() -> (w9:errorcluster)
      n77 = property on="PT2 Enabled?" class="Bool (strict)"() -> ("Value"=w13:bool)  [unwired: 2 in, 2 out]
      n78 = property on="PT2 Bauds" class="DigNum (strict)"() -> ("Value"=w12:u32)  [unwired: 2 in, 2 out]
      n79 = property on="PT2 Address" class="DigNum (strict)"() -> ("Value"=w14:u8)  [unwired: 2 in, 2 out]
      n80 = local read "MG port"() -> (w10:refnum<visa-resource-name>)
      n81 = local read "MG error"() -> (w15:errorcluster)
      n82 = property on="Enabled?" class="Bool (strict)"() -> ("Value"=w18:bool)  [unwired: 2 in, 2 out]
      n83 = while {
        tunnel: w6 -> [w33]
        tunnel: w14 -> [w32]
        tunnel: w13 -> [w23]
        tunnel: w12 -> [w29]
        shift-right: [w22] -> _
        shift-left: w9 -> [w28]
        stop <- w26 stop-if-true
        # "Pulse Tube 2"
        n84 = case shown="True" w23 {
          tunnel: [dbl[] [0.0, 0.0, 0.0, 0.0, 0.0, 0.0, 0.0, 0.0] w50] -> w34
          tunnel: w33 -> [_ w49]
          tunnel: w28 -> [w35 w48]
          tunnel: w32 -> [_ w47]
          tunnel: w29 -> [_ w42]
          tunnel: [w35 w41] -> w21
          frame False {
          }
          frame True {
            n85 = call "PT Read Status.vi"("error in (no error)"=w48, "Baud"=w42, "Slave Address"=w47, "Com Port #"=w49) -> ("error out"=w41:errorcluster, "Response"=w51:T19)
            n86 = call "PT Parse Response.vi"("Response"=w51) -> ("Oil temp"=w56:T20, "He temp"=w55:cluster{"[2]":dbl, "[2]":dbl, "[2]":dbl, dbl}, "Out water temp"=w54:T21, "In water temp"=w53:T22, "P_high"=→"P High":cluster{"[0]":dbl, "[0]":dbl, "[0]":dbl, dbl}, "Numeric"=w60:i32, "P_low"=→"P Low":cluster{"[1]":dbl, "[1]":dbl, "[1]":dbl, dbl}, "Average pressure"=w46:cluster{"Low":dbl, "High":dbl}, "Current"=w40:cluster{"Current":dbl, "Threshold":dbl}, "PT Error"=w52:i32)  [unwired: 1 in]
            "Oil" <- w56
            "Motor" <- w40
            "PT Status" <- w60
            "Water Out" <- w54
            "Water In" <- w53
            "Helium" <- w55
            "P_avg 2" <- w46
            n87 = property on="PT Error" class="DigNum (strict)"("Val(Sgnl)"=w52) -> ()  [unwired: 2 in, 2 out]
            n88 = Unbundle By Name(w53) -> ("Values[0]"=w43:dbl)
            n89 = Unbundle By Name(w54) -> ("[1]"=w59:dbl)
            n90 = Unbundle By Name(w55) -> ("[2]"=w58:dbl)
            n91 = Unbundle By Name(w56) -> ("[3]"=w57:dbl)
            n92 = Unbundle By Name(w46) -> ("Low"=w45:dbl, "High"=w44:dbl)
            n93 = Unbundle By Name(w40) -> ("Current"=w39:dbl)
            n94 = Not Equal To 0?(x=w60) -> (x != 0?=w61:bool)
            n95 = Boolean To (0,1)(Boolean=w61) -> (0, 1=w62:i16)
            n96 = Build Array(w62, w43, w59, w58, w57, w45, w44, w39) -> (w50:dbl[])
          }
        }
        n97 = property on="Averages" class="DigNum (strict)"() -> ("Value"=w31:i32)  [unwired: 2 in, 2 out]
        n98 = local read "Stop"() -> (w25:bool)
        n99 = call "Running average.vi"("Window Size"=w31, "New values"=w34) -> ("Filterred"=→"PT2 Data":dbl[])  [unwired: 2 in]
        n100 = call "MGI Clear Error.vi"("Error In"=w21) -> ("Error Out"=w22:errorcluster)  [unwired: 6 in]
        n101 = Not(x=w23) -> (.not. x?=w24:bool)
        n102 = local write "PT2 error"(w21) -> ()
        n103 = Or(x=w25, y=w24) -> (x .or. y?=w26:bool)
        n104 = Wait (ms)(milliseconds to wait=u32 250) -> ()  [unwired: 1 out]
      }
      n105 = while {
        tunnel: w18 -> [w123]
        shift-right: [w127] -> _
        shift-left: w15 -> [w126]
        shift-right: [w125] -> _
        shift-left: w10 -> [w128]
        stop <- w124 stop-if-true
        # "MaxiGauge"
        n106 = case shown="True" w123 {
          tunnel: w128 -> [w132 w136]
          tunnel: [w131 w135] -> w127
          tunnel: w126 -> [w131 w134]
          tunnel: [w132 w133] -> w125
          frame False {
          }
          frame True {
            n107 = case shown="No Error" w134 {
              selector: w134 -> [w143 _]
              tunnel: w136 -> [w151 w161]
              tunnel: [w137 w152] -> w135
              tunnel: [w150 w160] -> w133
              frame No Error {
                n108 = call "MG collect pressureinfo.vi"("error in"=w143, "MaxiGauge port"=w151) -> ("error out"=w148:T23, "sensor values"=w146:dbl[], "MaxiGauge port"=w142:refnum<visa-resource-name>, "sensor status info"=w141:string[])  [unwired: 4 in, 2 out]
                n109 = call "MG get errorstatus.vi"("error in"=w148, "MaxiGauge port"=w142) -> ("error out"=w138:T23, "MaxiGauge port"=w150:refnum<visa-resource-name>)  [unwired: 2 in, 2 out]
                n110 = property on="Averages" class="DigNum (strict)"() -> ("Value"=w145:i32)  [unwired: 2 in, 2 out]
                n111 = call "Running average.vi"("Window Size"=w145, "New values"=w146) -> ("Filterred"=w144:dbl[])  [unwired: 2 in]
                "MG Data" <- w144
                n112 = Array To Cluster(array=w141) -> (cluster=→"Sensors Status":T24)
                n113 = Array To Cluster(array=w144) -> (cluster=→"MG pressures":T25)
                n114 = call "Wait (ms)__ogtk.vi"("error in (no error)"=w138, "Wait on Error (FALSE)"=TRUE, "milliseconds to wait"=u32 500) -> ("error out"=w137:errorcluster)  [unwired: 7 in, 1 out]
              }
              frame Error {
                w156 = TRUE ("ID query")
                n115 = VISA Close(VISA resource name=w161) -> (error out=w159:errorcluster)  [unwired: 1 in]
                n116 = call "VISA Check port.vi"("error in (no error)"=w159, "VISA Resource Name in"=w161) -> ("error out"=w158:errorcluster, "VISA Resource Name out"=w157:refnum<visa-resource-name>)  [unwired: 8 in]
                n117 = call "MG initialize.vi"("error in (no error)"=w158, "MG query errorstatus"=w156, "ID query"=w156, "MaxiGauge port"=w157) -> ("error out"=w153:errorcluster, "MaxiGauge port"=w160:refnum<visa-resource-name>)  [unwired: 2 in, 1 out]
                n118 = call "Wait (ms)__ogtk.vi"("error in (no error)"=w153, "Wait on Error (FALSE)"=TRUE, "milliseconds to wait"=u32 1000) -> ("error out"=w152:errorcluster)  [unwired: 7 in, 1 out]
              }
            }
          }
        }
        n119 = local read "Stop"() -> (w129:bool)
        n120 = Not(x=w123) -> (.not. x?=w122:bool)
        n121 = Or(x=w122, y=w129) -> (x .or. y?=w124:bool)
        n122 = local write "MG error"(w127) -> ()
        n123 = Wait (ms)(milliseconds to wait=u32 500) -> ()  [unwired: 1 out]
      }
    }
    frame #2 {
      n124 = Set Occurrence(w204) -> ()
    }
  }
  n125 = while {
    shift-right: [w212] -> _
    shift-left: w2 -> [w218]
    shift-right: [w216] -> _
    shift-left: w2 -> [w217]
    tunnel: w4 -> [w215]
    shift-right: [w213] -> _
    shift-left: w1 -> [w214]
    shift-right: [w209] -> _
    shift-left: w2 -> [w211]
    shift-right: [w208] -> _
    shift-left: w2 -> [w210]
    tunnel: w3 -> [w207]
    shift-right: [w205] -> _
    shift-left: w1 -> [w206]
    stop <- w220 stop-if-true
    n126 = event shown="[0] Timeout" {
      selector: _ -> [_ _ _ _ _ _ _ _ _ _ _ _ _ _ _ _ _ _ _ _ _ _ _ _ _ _ _ _ _ _ _]
      dyn-events: _ -> [_ _ _ _ _ _ _ _ _ _ _ _ _ _ _ _ _ _ _ _ _ _ _ _ _ _ _ _ _ _ _]
      timeout: 250 -> [_ _ _ _ _ _ _ _ _ _ _ _ _ _ _ _ _ _ _ _ _ _ _ _ _ _ _ _ _ _ _]
      tunnel: [_ _ TRUE _ _ _ _ _ _ _ _ _ _ _ _ _ _ _ _ _ _ _ _ _ _ _ _ _ _ _ _] -> w220
      tunnel: w218 -> [w221 w466 w632 w664 w673 w682 w691 w703 w734 w743 w749 w762 w776 w780 w885 w894 w907 w923 w938 w944 w964 w974 w989 w996 w1004 w1012 w1023 w1040 w1046 w1069 w1074]
      tunnel: w217 -> [w224 w468 w631 w663 w672 w681 w690 w702 w733 w742 w747 w760 w774 w784 w884 w893 w908 w922 w937 w943 w963 w973 w988 w997 w1005 w1011 w1022 w1039 w1044 w1068 w1077]
      tunnel: [w224 w467 w618 w663 w672 w681 w690 w702 w733 w742 w747 w760 w774 w784 w884 w893 w906 w922 w937 w943 w963 w973 w988 w997 w1005 w1011 w1022 w1039 w1044 w1068 w1077] -> w216
      tunnel: w215 -> [_ w464 _ _ _ _ _ _ _ _ _ _ _ _ _ _ _ _ _ _ _ _ _ _ _ _ _ _ _ _ _]
      tunnel: w214 -> [w227 w456 _ w662 w671 w680 w689 w699 w732 w741 w755 w767 w778 w783 w883 w895 _ w924 w936 w945 w962 w975 w985 w995 w1003 w1013 w1024 w1038 w1045 w1067 w1079]
      tunnel: [w227 w458 w617 w662 w671 w680 w689 w699 w732 w741 w755 w767 w778 w783 w883 w895 w896 w924 w936 w945 w962 w975 w985 w995 w1003 w1013 w1024 w1038 w1045 w1067 w1079] -> w213
      tunnel: [w222 w465 w618 w664 w673 w682 w691 w703 w734 w743 w748 w761 w775 w779 w885 w894 w909 w923 w938 w944 w964 w974 w989 w996 w1004 w1012 w1023 w1040 w1046 w1069 w1073] -> w212
      tunnel: w211 -> [w226 w463 w630 w661 w670 w679 w688 w695 w731 w740 w746 w759 w773 w782 w882 w892 w905 w921 w934 w942 w961 w972 w987 w999 w1006 w1010 w1021 w1036 w1043 w1065 w1076]
      tunnel: w210 -> [w225 w462 w629 w660 w669 w678 w687 w694 w730 w739 w745 w758 w772 w781 w881 w891 w903 w920 w933 w941 w960 w971 w986 w998 w1007 w1009 w1020 w1035 w1042 w1064 w1075]
      tunnel: [w226 w461 w618 w661 w670 w679 w688 w695 w731 w740 w746 w759 w773 w782 w882 w892 w904 w921 w934 w942 w961 w972 w987 w993 w1006 w1010 w1021 w1036 w1043 w1065 w1076] -> w209
      tunnel: [w225 w460 w618 w660 w669 w678 w687 w694 w730 w739 w745 w758 w772 w781 w881 w891 w902 w920 w933 w941 w960 w971 w986 w998 w1001 w1009 w1020 w1035 w1042 w1064 w1075] -> w208
      tunnel: w207 -> [_ _ w628 _ _ _ _ _ _ _ _ _ _ _ _ _ _ _ _ _ _ _ _ _ _ _ _ _ _ _ _]
      tunnel: w206 -> [w223 w459 _ w659 w668 w677 w686 w693 w729 w738 w754 w768 w777 w786 w880 w890 _ w911 w935 w940 w950 w967 w984 w992 w1000 w1008 w1019 w1037 w1041 w1066 w1078]
      tunnel: [w223 w457 w617 w659 w668 w677 w686 w693 w729 w738 w754 w768 w777 w786 w880 w890 w898 w911 w935 w940 w950 w967 w984 w992 w1000 w1008 w1019 w1037 w1041 w1066 w1078] -> w205
      event Timeout {
        n127 = First Call?() -> (First Call?: T/F=w228:bool)
        n128 = event-data() -> ()  [unwired: 1 in, 3 out]
        n129 = case shown="False" w228 {
          tunnel: w221 -> [w230 w395]
          tunnel: [w229 w395] -> w222
          frame False {
            n130 = stacked-sequence {
              tunnel: w230 -> [_ _ _ w355]
              tunnel: [_ _ _ w354] -> w229
              frame #0 {
                n131 = Unbundle By Name("Log Options") -> ("Every  2"=w247:dbl, "Save to log"=w248:bool, "Every1"=w238:dbl, "Plot data"=w249:bool)
                n132 = local read "ForceSave"() -> (w239:bool)
                n133 = local read "FP Status bits"() -> (w234:u32[])
                n134 = call "Time Elapsed.vi"("Every"=w247, "Time Units"=enum16{"Minutes", "Hours", "Days"}."Minutes") -> ("Triggered?"=w243:bool)  [unwired: 1 in]
                n135 = local read "PT1 Data"() -> (w233:dbl[])
                n136 = local read "PT2 Data"() -> (w237:dbl[])
                n137 = local read "MG Data"() -> (w232:dbl[])
                n138 = call "Time Elapsed.vi"("Every"=w238, "Time Units"=enum16{"Minutes", "Hours", "Days"}."Minutes") -> ("Triggered?"=w242:bool)  [unwired: 1 in]
                n139 = local read "FP Data"() -> (w231:sgl[])
                n140 = Or(x=w239, y=w243) -> (x .or. y?=w241:bool)
                n141 = Or(x=w239, y=w242) -> (x .or. y?=w240:bool)
                n142 = And(x=w240, y=w249) -> (x .and. y?=w260:bool)
                n143 = And(x=w241, y=w248) -> (x .and. y?=w261:bool)
                n144 = case shown="True" w261 {
                  tunnel: w231 -> [_ w288]
                  tunnel: w232 -> [_ w301]
                  tunnel: w234 -> [_ w300]
                  tunnel: w233 -> [_ w302]
                  tunnel: "Log Options" -> [_ w295]
                  tunnel: w239 -> [_ _]
                  tunnel: w237 -> [_ w282]
                  frame False {
                  }
                  frame True {
                    n145 = Unbundle By Name(w295) -> ("Filename suffix"=w292:string, "AVS_Path 2"=w294:path, "AVS_FName"=w293:string, "NewFevery"=w286:u32, "Time Units"=w285:enum16{"Minutes", "Hours", "Days"}, "Date Format"=w284:string)
                    n146 = call "Combine Data 4 logging.vi"("FP Status Bits"=w300, "Time Format String"=w284, "PT2 Data"=w282, "PT1 Data"=w302, "MG Data"=w301, "FP Data"=w288) -> ("Array"=w291:string[])  [unwired: 1 in]
                    n147 = local read "Cur Path"() -> (w289:path)
                    n148 = call "Format header.vi"("FP Data"=w288) -> ("Header string"=w287:string)  [unwired: 4 in]
                    n149 = call "File Date.vi"("Cur Path"=w289) -> ("Time Stamp"=w299:timestamp)  [unwired: 4 in]
                    n150 = call "Time Elapsed time.vi"("Time Units"=w285, "Delay Time"=w286, "Time Old In"=w299) -> ("T>dT?"=w290:bool)  [unwired: 2 out]
                    n151 = case shown="True" w290 {
                      tunnel: [w304 w306] -> w297
                      tunnel: [_ w310] -> w296
                      tunnel: w294 -> [_ w309]
                      tunnel: w293 -> [_ w308]
                      tunnel: w292 -> [_ w307]
                      tunnel: w289 -> [w304 _]
                      tunnel: w287 -> [_ w305]
                      frame False {
                      }
                      frame True {
                        n152 = call "GeneratePaths.vi"("Filename Suffix"=w307, "AVS_Path"=w309, "AVS_FName"=w308) -> ("Generated Log path"=w306:path)  [unwired: 11 in, 1 out]
                        n153 = Write to Text File(file (use dialog)=w306, text=w305) -> (error out=w310:errorcluster)  [unwired: 2 in, 2 out]
                      }
                    }
                    n154 = call "Write To Spreadsheet File (string) w Error.vi"("append to file? (new file:F)"=TRUE, "error in"=w296, "1D data"=w291, "file path (dialog if empty)"=w297) -> ("new file path (Not A Path if cancelled)"=→"Cur Path":path)  [unwired: 6 in, 1 out]
                    n155 = local write "ForceSave"(FALSE ("ForceSave")) -> ()
                  }
                }
                n156 = case shown="True" w260 {
                  tunnel: w232 -> [_ w271]
                  tunnel: w231 -> [_ w281]
                  tunnel: w233 -> [_ w272]
                  tunnel: w237 -> [_ w265]
                  frame False {
                  }
                  frame True {
                    w264 = 1 ("Smoothing window")
                    n157 = Get Date/Time In Seconds() -> (seconds since 1Jan1904=w280:timestamp)
                    n158 = To Double Precision Float(number=w280) -> (double precision float=w279:dbl)
                    n159 = call "AppendData1.vi"("Smoothing window"=w264, "Current Measurement"=w279) -> ("Data Out"=w262:dbl[])  [unwired: 4 in]
                    n160 = call "AppendData.vi"("Smoothing window"=w264, "Current Measurement"=w265) -> ("Data Out"=w263:sgl[][])  [unwired: 4 in]
                    n161 = call "AppendData.vi"("Smoothing window"=w264, "Current Measurement"=w281) -> ("Data Out"=w267:sgl[][])  [unwired: 4 in]
                    n162 = call "AppendData.vi"("Smoothing window"=w264, "Current Measurement"=w271) -> ("Data Out"=w268:sgl[][])  [unwired: 4 in]
                    n163 = call "AppendData.vi"("Smoothing window"=w264, "Current Measurement"=w272) -> ("Data Out"=w269:sgl[][])  [unwired: 4 in]
                    n164 = call "MultiRPlot_Select1.vi"("Time"=w262, "FP Plots Select"="FP Plots Select", "Data In"=w267) -> ("Out Array"=→"Front Panel":cluster{"Time":dbl[], "Value":dbl[]}[])  [unwired: 1 in]
                    n165 = call "MultiRPlot_Select1.vi"("Time"=w262, "FP Plots Select"="MG Plots Select", "Data In"=w268) -> ("Out Array"=→"MaxiGauge":cluster{"Time":dbl[], "Value":dbl[]}[])  [unwired: 1 in]
                    n166 = call "MultiRPlot_Select1.vi"("Time"=w262, "FP Plots Select"="PT1 Plots Select", "Data In"=w269) -> ("Out Array"=→"PT1 Status 2":cluster{"Time":dbl[], "Value":dbl[]}[])  [unwired: 1 in]
                    n167 = call "MultiRPlot_Select1.vi"("Time"=w262, "FP Plots Select"="PT2 Plots Select", "Data In"=w263) -> ("Out Array"=→"PT2 Status":cluster{"Time":dbl[], "Value":dbl[]}[])  [unwired: 1 in]
                  }
                }
                n168 = Array To Cluster(array=w231) -> (cluster=w259:T27)
                n169 = property on="P8" class="Ring (strict)"() -> ("Value"=w257:u16)  [unwired: 2 in, 2 out]
                n170 = Unbundle(w259) -> ("FP Data[0]"=→"P1" →"P1":sgl, "FP Data[1]"=→"P2" →"P2":sgl, "FP Data[2]"=→"P3" →"P3":sgl, "FP Data[3]"=→"P4" →"P4":sgl, "FP Data[4]"=→"P5" →"P5":sgl, "FP Data[5]"=→"P6" →"4He":sgl, "FP Data[6]"=→"P7" →"3He":sgl, "FP Data[7]"=→"Flow" →"FLOW":sgl, "FP Data[8]"=→"PC" →"PC":sgl)
                n171 = Index Array(array=w232, index=w257) -> (element=→"Pstill (P8)":dbl)
              }
              frame #1 {
                n172 = local read "Mode"() -> (w312:u16)
                n173 = local read "FP Status bits"() -> (w313:u32[])
                n174 = local read "PT1 Data"() -> (w317:dbl[])
                n175 = local read "MG Data"() -> (w316:dbl[])
                n176 = local read "FP Data"() -> (w315:sgl[])
                n177 = Bundle By Name(cluster=T26 {"FP Data"=[], "MG Data"=[], "PT Data"=[], "FP Status Bits"=[], "Mode"=0} ("FP cluster"), "FP Data"=w315, "MG Data"=w316, "PT Data"=w317, "FP Status Bits"=w313, "Mode"=w312) -> (w314:T26)
                n178 = call "FP_to_DSC.vi"("FP cluster"=w314) -> ()  [unwired: 10 in, 1 out]
              }
              frame #2 {
                # "Check if the structure is \nnot empty and only one\nof Scalar or Array controls \nis set"
                # "Set FP control value from external script/program"
                n179 = local read "SetControl"() -> (w329:T7)
                n180 = Unbundle By Name(w329) -> ("Name"=w327:string, "Scalar"=w328:string, "Array"=w319:string[][])
                n181 = call "Empty 2D Array (String)__ogtk.vi"("Array"=w319) -> ("Empty Array?"=w322:bool)  [unwired: 8 in]
                n182 = Empty String/Path?(string/path=w327) -> (empty?=w323:bool)
                n183 = Empty String/Path?(string/path=w328) -> (empty?=w324:bool)
                n184 = Not(x=w323) -> (.not. x?=w325:bool)
                n185 = Not(x=w324) -> (.not. x?=w321:bool)
                n186 = Not(x=w322) -> (.not. x?=w318:bool)
                n187 = Exclusive Or(1:w318, 2:w321) -> (0:w320:bool)
                n188 = And(x=w325, y=w320) -> (x .and. y?=w326:bool)
                n189 = case shown="False" w326 {
                  tunnel: w327 -> [_ w333]
                  tunnel: w328 -> [_ w332]
                  tunnel: w319 -> [_ w331]
                  tunnel: w318 -> [_ w330]
                  frame False {
                  }
                  frame True {
                    n190 = flat-sequence {
                      tunnel: w333 -> [w337]
                      tunnel: w332 -> [w336]
                      tunnel: w331 -> [w334]
                      tunnel: w330 -> [w335]
                      frame #0 {
                        n191 = local read "VIRef"() -> (w338:T1)
                        n192 = case shown="True" w335 {
                          tunnel: w338 -> [w341 w344]
                          tunnel: w337 -> [w340 w343]
                          tunnel: w336 -> [w339 _]
                          tunnel: w334 -> [_ w342]
                          frame False {
                            n193 = call "Push2VI.vi"("New Value"=w339, "element"=w340, "VIRef"=w341) -> ()  [unwired: 8 in, 1 out]
                          }
                          frame True {
                            n194 = call "PushArray2VI.vi"("Str"=w342, "element"=w343, "VIRef"=w344) -> ()  [unwired: 8 in, 1 out]
                          }
                        }
                      }
                      frame #1 {
                        w346 = ""
                        # "Empty the cluster to flag that\nthe command is processed"
                        n195 = Bundle(w346, w346, "Array"=string[][] []) -> (→"SetControl":cluster{string, string, "Array":string[][]})  [unwired: 1 in]
                      }
                    }
                  }
                }
              }
              frame #3 {
                n196 = local read "MG error"() -> (w352:errorcluster)
                n197 = local read "FP error"() -> (w353:errorcluster)
                n198 = Not(x=w353) -> (.not. x?=w351:bool)
                n199 = Not(x=w352) -> (.not. x?=w350:bool)
                n200 = Compound Arithmetic op=AND(w351, w350, "EnableAutoCond") -> (w348:bool)
                n201 = case shown="True" w348 {
                  tunnel: w355 -> [w356 w372]
                  tunnel: [w356 w371] -> w354
                  frame False {
                    n202 = call "MGI Milliseconds Since Last Reset.vi"("Reset (F)"=TRUE) -> ()  [unwired: 5 in, 2 out]
                  }
                  frame True {
                    n203 = local read "MG Data"() -> (w379:dbl[])
                    n204 = Index Array(array=w379, index="MG  channel") -> (element=w377:dbl)
                    n205 = Not(x="Cond2") -> (.not. x?=w373:bool)
                    n206 = Less?(x=w377, y="P threshold") -> (x < y?=w375:bool)
                    n207 = Or(x=w375, y=w373) -> (x .or. y?=w359:bool)
                    "SP reached? 3" <- w359
                    n208 = Not(x=w359) -> (.not. x?=w361:bool)
                    n209 = call "MGI Milliseconds Since Last Reset.vi"("Reset (F)"=w361) -> ("ms"=w370:u32)  [unwired: 5 in, 1 out]
                    n210 = Divide(x=w370, y=u32 1000) -> (x/y=w367:dbl)
                    "Delay Timer" <- w367
                    n211 = Multiply(x="Delay Time", y=u32 60) -> (x*y=w363:u32)
                    n212 = Not(x="Cond1") -> (.not. x?=w364:bool)
                    n213 = Greater Or Equal?(x=w367, y=w363) -> (x >= y?=w366:bool)
                    n214 = Or(x=w366, y=w364) -> (x .or. y?=w360:bool)
                    "SP reached? 2" <- w360
                    n215 = And(x=w359, y=w360) -> (x .and. y?=w358:bool)
                    "SP reached?" <- w358
                    n216 = case shown="True" w358 {
                      tunnel: w372 -> [w380 w382]
                      tunnel: [w380 w381] -> w371
                      frame False {
                      }
                      frame True {
                        # "Auto"
                        # "Start"
                        # "Reset"
                        n217 = call "BP togglekey.vi"("keynumber"=u16 10, "FrontPanel port"=w382) -> ("error out"=w394:T18, "FrontPanel port"=w389:refnum<visa-resource-name>)  [unwired: 2 in]
                        n218 = local write "EnableAutoCond"(FALSE ("EnableAutoCond")) -> ()
                        n219 = call "MGI Wait (U32).vi"("ms"=u32 2000, "Error In"=w394) -> ("Error Out"=w393:errorcluster)  [unwired: 5 in]
                        n220 = call "BP togglekey.vi"("error in"=w393, "keynumber"=u16 48, "FrontPanel port"=w389) -> ("error out"=w392:T18, "FrontPanel port"=w391:refnum<visa-resource-name>)  [unwired: 1 in]
                        n221 = call "MGI Wait (U32).vi"("ms"=u32 500, "Error In"=w392) -> ("Error Out"=w390:errorcluster)  [unwired: 5 in]
                        n222 = call "BP togglekey.vi"("error in"=w390, "keynumber"=u16 54, "FrontPanel port"=w391) -> ("FrontPanel port"=w381:refnum<visa-resource-name>)  [unwired: 1 in, 1 out]
                      }
                    }
                  }
                }
              }
            }
          }
          frame True {
            n223 = stacked-sequence {
              frame #0 {
                w403 = T28."Page Disabled & Grayed" ("Page Enabled State")
                w404 = u8 2 ("Disabled")
                w416 = u8 1 ("Disabled")
                w420 = u32 16777062
                w425 = u32 65382
                w424 = u32 0
                w423 = 0.1
                w422 = 2000
                w421 = 0
                n224 = property class="App"() -> ("App.Kind"=w426:T29)  [unwired: 2 in, 2 out]
                n225 = property on="Hide side panel" class="Bool (strict)"("Val(Sgnl)"=FALSE ("Value (Signaling)")) -> ()  [unwired: 2 in, 2 out]
                n226 = property on="S1" class="TabCtl (strict)"("Disabled"=w404) -> ()  [unwired: 2 in, 2 out]
                n227 = property on="S2" class="TabCtl (strict)"("Disabled"=w404) -> ()  [unwired: 2 in, 2 out]
                n228 = property on="Stop" class="Bool (strict)"("Disabled"=w404) -> ()  [unwired: 2 in, 2 out]
                n229 = property on="Error panel" class="TabCtl (strict)"("Disabled"=w404) -> ()  [unwired: 2 in, 2 out]
                n230 = property on="Main Panel" class="TabCtl (strict)"("Disabled"=w404) -> ()  [unwired: 2 in, 2 out]
                n231 = property on="Main Panel" class="TabCtl (strict)"("Disabled"=w404) -> ()  [unwired: 2 in, 2 out]
                n232 = call "Current VIs Reference__ogtk.vi"() -> ("Current VI's reference"=w410:refnum<vi>)  [unwired: 5 in]
                n233 = case shown="\"invalid app kind\", Default" w426 {
                  tunnel: [w428 w437] -> w427
                  frame "invalid app kind", Default {
                    n234 = control-ref of="This VI"() -> (w429:refnum<vi>)
                    n235 = property class="VI"(reference=w429) -> ("Hist.Revision"=w430:u32)  [unwired: 1 in, 2 out]
                    n236 = Divide(x=w430, y=1000.0 ("x")) -> (x/y=w434:dbl)
                    n237 = Number To Fractional String(use system decimal point (T)=FALSE, number=w434, precision (6)=i16 2) -> (F-format string=w435:string)  [unwired: 1 in]
                    n238 = Concatenate Strings("" ("string"), w435) -> (w428:string)
                  }
                  frame "Run Time System" {
                    n239 = Current VI's Path() -> (path=w440:path)
                    n240 = Strip Path(path=w440) -> (stripped path=w441:path)  [unwired: 1 out]
                    n241 = Path To String(path=w441) -> (string=w439:string)
                    n242 = invoke class="FileVersionInfo" method="GetVersionInfo"("fileName"=w439) -> ("GetVersionInfo"=w438:refnum<k24>)  [unwired: 3 in, 3 out]
                    n243 = property class="FileVersionInfo"(reference=w438) -> ("FileVersion"=w437:string)  [unwired: 1 in, 2 out]
                  }
                }
                "V" <- w427
                n244 = local write "Cur Path"(path "") -> ()
                n245 = call "GetFrontPanelControls.vi"("Ref to VI"=w410) -> ("VIRef"=w411:T1)  [unwired: 9 in, 1 out]
                "VIRef" <- w411
                n246 = Unbundle By Name(w411) -> ("Full Name"=→"ControlNames":string[])
                n247 = call "Current VI's Path__ogtk.vi"() -> ("Current VI's Path (+ Relative)"=w397:path)  [unwired: 1 in]
                n248 = property on="Side Panel" class="TabCtl (strict)"("Value"=enum32{"Main", "Settings", "Advanced"}."Settings" ("Side Panel")) -> ("Pages"=w400:refnum<vi>[])  [unwired: 2 in, 2 out]
                n249 = Path To String(path=w397) -> (string=→"VI path":string)
                n250 = Index Array(array=w400) -> (element #1=w401:refnum<vi>, element #3=w402:refnum<vi>)  [unwired: 3 in, 1 out]
                n251 = property class="Page"(reference=w401, "PageEnb"=w403) -> ()  [unwired: 1 in, 2 out]
                n252 = property class="Page"(reference=w402, "PageEnb"=w403) -> ()  [unwired: 1 in, 2 out]
                n253 = property on="3He" class="Slide (strict)"("Scale.Range:Minimum"=w421, "Scale.Range:Maximum"=w422, "Scale.Range:Increment"=w423) -> ()  [unwired: 2 in, 2 out]
                n254 = property on="P1" class="DigNum (strict)"("Numeric Text.Text Colors:Text Color"=w424, "Numeric Text.Text Colors:BG Color"=w420) -> ()  [unwired: 2 in, 2 out]
                n255 = property on="P4" class="DigNum (strict)"("Numeric Text.Text Colors:Text Color"=w424, "Numeric Text.Text Colors:BG Color"=w425) -> ()  [unwired: 2 in, 2 out]
                n256 = Initialize Array(FALSE, 64 ("dimension size")) -> (w396:bool[])
                n257 = property on="Start" class="Bool (strict)"("Visible"=TRUE, "Disabled"=u8 0) -> ()  [unwired: 2 in, 2 out]
                n258 = control-ref of="LEDs"() -> (w407:refnum<vi>)
                n259 = call "FP Set Binking Controls.vi"("Cluster in"=w407, "Array of blinking states"=w396, "Array of relais states"=w396) -> ()  [unwired: 13 in]
                n260 = property on="P2" class="DigNum (strict)"("Numeric Text.Text Colors:Text Color"=w424, "Numeric Text.Text Colors:BG Color"=w420) -> ()  [unwired: 2 in, 2 out]
                n261 = property on="P5" class="DigNum (strict)"("Numeric Text.Text Colors:Text Color"=w424, "Numeric Text.Text Colors:BG Color"=w425) -> ()  [unwired: 2 in, 2 out]
                n262 = property on="4He" class="Slide (strict)"("Scale.Range:Minimum"=w421, "Scale.Range:Maximum"=w422, "Scale.Range:Increment"=w423) -> ()  [unwired: 2 in, 2 out]
                n263 = control-ref of="LEDs 2"() -> (w408:refnum<vi>)
                n264 = property on="Configuration" class="Clust (strict)"("Disabled"=u8 0) -> ()  [unwired: 2 in, 2 out]
                n265 = call "FP Set Binking Controls.vi"("Cluster in"=w408, "Array of blinking states"=w396, "Array of relais states"=w396) -> ()  [unwired: 13 in]
                n266 = local write "EnableAutoCond"(FALSE ("EnableAutoCond")) -> ()
                n267 = property on="P3" class="DigNum (strict)"("Numeric Text.Text Colors:Text Color"=w424, "Numeric Text.Text Colors:BG Color"=w420) -> ()  [unwired: 2 in, 2 out]
                n268 = property on="FLOW" class="DigNum (strict)"("Numeric Text.Text Colors:Text Color"=w424, "Numeric Text.Text Colors:BG Color"=w425) -> ()  [unwired: 2 in, 2 out]
                n269 = property on="Panel ID" class="Str"("Text.Text Colors:Text Color"=u32 13311) -> ()  [unwired: 2 in, 2 out]
                n270 = property on="Buttons" class="Clust"("Disabled"=w416) -> ()  [unwired: 2 in, 2 out]
                n271 = property on="Buttons 2" class="Clust"("Disabled"=w416) -> ()  [unwired: 2 in, 2 out]
              }
              frame #1 {
                # "First load the settings from the old location then \nfrom the new one. This way the program will \"transfer\" \nthe settings to the new config file after the upgrade"
                n272 = call "Create Dir if Non-Existant__ogtk.vi"("Directory Path"=path "C:/LC Data/Configuration/FP" ("Relative path (.)")) -> ("dup Directory Path"=w444:path)  [unwired: 8 in, 2 out]
                n273 = call "Build Path - Traditional__ogtk.vi"("name or relative path"="FP config.ini", "base path"=w444) -> ("appended path"=w442:path)
                n274 = control-ref of="Configuration"() -> (w454:refnum<vi>)
                n275 = control-ref of="ADC scaling"() -> (w451:refnum<vi>)
                n276 = control-ref of="Log Options"() -> (w450:refnum<vi>)
                n277 = call "Current VIs Parent Directory__ogtk.vi"("Relative path (.)"=path "config.ini") -> ("Parent Directory (+ Relative)"=w452:path)  [unwired: 4 in]
                n278 = Build Array(w454, w451, w450) -> (w447:refnum<vi>[])
                n279 = call "Save Load Settings to File by Ref with path.vi"("Array of Cluster References"=w447, "Action"=enum8{"Load", "Save"}."Load", "Configuration file"=w452) -> ("error out"=w448:errorcluster)  [unwired: 6 in]
                n280 = call "MGI Clear Error.vi"("Error In"=w448) -> ("Error Out"=w449:errorcluster)  [unwired: 6 in]
                n281 = call "Save Load Settings to File by Ref with path.vi"("Array of Cluster References"=w447, "Action"=enum8{"Load", "Save"}."Load", "error in (no error)"=w449, "Configuration file"=w442) -> ()  [unwired: 5 in, 1 out]
              }
            }
          }
        }
      }
      event "Start": Value Change {
        n282 = event-data() -> ()  [unwired: 1 in, 6 out]
        n283 = stacked-sequence {
          tunnel: w468 -> [_ w518 _ _ _ _]
          tunnel: [_ w517 _ _ _ _] -> w467
          tunnel: w466 -> [w483 _ _ _ _ _]
          tunnel: [w470 _ _ _ _ _] -> w465
          tunnel: w464 -> [_ _ _ _ _ w616]
          tunnel: w463 -> [_ _ _ w589 _ _]
          tunnel: w462 -> [_ _ _ w588 _ _]
          tunnel: [_ _ _ w586 _ _] -> w461
          tunnel: [_ _ _ w587 _ _] -> w460
          tunnel: w456 -> [_ _ _ _ _ _]
          tunnel: w459 -> [_ _ _ _ _ _]
          tunnel: [_ _ w544 _ _ _] -> w458
          tunnel: [_ _ w548 _ _ _] -> w457
          frame #0 {
            n284 = call "Stop Display Busy AE.vi"("Action"=enum16{"Write", "Read"}."Write", "Error In"=T18 {"error"=FALSE, "code"=0, "source"=""} ("error in"), "Stop?"=FALSE) -> ("Error Out"=w471:errorcluster)  [unwired: 7 in, 1 out]
            n285 = property on="FP baud rate" class="DigNum (strict)"() -> ("Value"=w482:u32)  [unwired: 2 in, 2 out]
            n286 = call "FP-Scan ports.vi"("Error in"=w471, "baud rate"=w482, "RS232 port"=w483) -> ("Error out"=w474:errorcluster, "ID string"=w480:string, "VISA Refnum out"=w481:refnum<visa-resource-name>)  [unwired: 5 in, 1 out]
            "Panel ID" <- w480
            n287 = call "Stop Display Busy AE.vi"("Action"=enum16{"Write", "Read"}."Write", "Error In"=w474, "Stop?"=TRUE) -> ("Error Out"=w473:errorcluster)  [unwired: 7 in, 1 out]
            n288 = call "Get GHS version and type.vi"("ID string"=w480, "error in (no error)"=w473) -> ("Panel Version"=w488:bool, "System Type"=w487:bool, "error out"=w484:errorcluster)  [unwired: 4 in]
            n289 = call "Display Busy.vi"("error in (no error)"=w471, "Title"="Trying to connect to the Front Panel") -> ()  [unwired: 8 in, 2 out]
            n290 = Boolean To (0,1)(Boolean=w488) -> (0, 1=w469:i16)
            n291 = Boolean To (0,1)(Boolean=w487) -> (0, 1=w486:i16)
            n292 = property on="FP Layout" class="TabCtl (strict)"("Value"=w469) -> ()  [unwired: 2 in, 2 out]
            n293 = property on="Panel Layout" class="Enum (strict)"("Value"=w469) -> ()  [unwired: 2 in, 2 out]
            n294 = property on="Type" class="RadioBtnsControl (strict)"("Val(Sgnl)"=w486) -> ()  [unwired: 2 in, 2 out]
            n295 = call "BP query settings.vi"("error in"=w484, "FrontPanel port"=w481) -> ("error out"=w485:T18, "array of 4 x 16 bit unsigned"=w495:u16[], "FrontPanel port"=w496:refnum<visa-resource-name>)  [unwired: 2 in, 1 out]
            "FP error" <- w485
            n296 = call "BP query P5.vi"("error in"=w485, "FrontPanel port"=w496) -> ("error out"=w509:T18, "array of 2 x 16 bit unsigned"=w514:u16[], "FrontPanel port"=w515:refnum<visa-resource-name>)  [unwired: 2 in, 1 out]
            n297 = Array To Cluster(array=w495) -> (cluster=w494:T30)
            n298 = Array To Cluster(array=w514) -> (cluster=w507:T31)
            n299 = call "Disable on error.vi"("error out"=w509) -> ("Numeric"=w510:i16)
            n300 = property on="P6&7 limits" class="Clust (strict)"("Value"=w494) -> ()  [unwired: 2 in, 2 out]
            n301 = call "BP query NCP5.vi"("error in"=w485, "FrontPanel port"=w515) -> ("error out"=w512:T18, "array of 3 x 16 bit unsigned"=w513:u16[], "FrontPanel port"=w506:refnum<visa-resource-name>)  [unwired: 2 in, 1 out]
            n302 = property on="P5 Settings" class="Clust (strict)"("Value"=w507, "Disabled"=w510) -> ()  [unwired: 2 in, 2 out]
            n303 = Array To Cluster(array=w513) -> (cluster=w508:T32)
            n304 = call "Disable on error.vi"("error out"=w512) -> ("Numeric"=w511:i16)
            n305 = call "BP query NCP5B.vi"("error in"=w485, "FrontPanel port"=w506) -> ("error out"=w503:T18, "array of 3 x 16 bit unsigned"=w504:u16[], "FrontPanel port"=w505:refnum<visa-resource-name>)  [unwired: 2 in, 1 out]
            n306 = property on="NCP5 Settings" class="Clust (strict)"("Value"=w508, "Disabled"=w511) -> ()  [unwired: 2 in, 2 out]
            n307 = Array To Cluster(array=w504) -> (cluster=w501:cluster{"array of 3 x 16 bit unsigned[0]":u16})
            n308 = property on="P6&7 Settings" class="Clust (strict)"("Value"=w494) -> ()  [unwired: 2 in, 2 out]
            n309 = call "Disable on error.vi"("error out"=w503) -> ("Numeric"=w502:i16)
            n310 = call "BP Query REC.vi"("error in"=w485, "FrontPanel port"=w505) -> ("error out"=w499:T18, "array of 3 x 16 bit unsigned"=w500:u16[], "FrontPanel port"=w493:refnum<visa-resource-name>)  [unwired: 2 in, 1 out]
            n311 = property on="P5 limits" class="Clust (strict)"("Value"=w507) -> ()  [unwired: 2 in, 2 out]
            n312 = property on="NCP5B Settings" class="Clust (strict)"("Value"=w501, "Disabled"=w502) -> ()  [unwired: 2 in, 2 out]
            n313 = Array To Cluster(array=w500) -> (cluster=w497:T32)
            n314 = call "Disable on error.vi"("error out"=w499) -> ("Numeric"=w498:i16)
            n315 = call "BP Query Turbo.vi"("error in"=w485, "FrontPanel port"=w493) -> ("error out"=w491:T18, "array of 3 x 16 bit unsigned"=w490:u16[], "FrontPanel port"=w470:refnum<visa-resource-name>)  [unwired: 2 in, 1 out]
            "FP port" <- w470
            n316 = property on="REC Settings" class="Clust (strict)"("Value"=w497, "Disabled"=w498) -> ()  [unwired: 2 in, 2 out]
            n317 = property on="NCP5 limits" class="Clust (strict)"("Value"=w508) -> ()  [unwired: 2 in, 2 out]
            n318 = Array To Cluster(array=w490) -> (cluster=w489:cluster{"array of 3 x 16 bit unsigned[0]":u16})
            n319 = call "Disable on error.vi"("error out"=w491) -> ("Numeric"=w492:i16)
            n320 = property on="S1&2 Settings" class="Clust (strict)"("Value"=w489, "Disabled"=w492) -> ()  [unwired: 2 in, 2 out]
            n321 = property on="NCP5B limits" class="Clust (strict)"("Value"=w501) -> ()  [unwired: 2 in, 2 out]
            n322 = property on="REC limits" class="Clust (strict)"("Value"=w497) -> ()  [unwired: 2 in, 2 out]
            n323 = property on="FP port number" class="VISAName"("Value"=w470) -> ()  [unwired: 2 in, 2 out]
            n324 = property on="S1&2 limits" class="Clust (strict)"("Value"=w489) -> ()  [unwired: 2 in, 2 out]
          }
          frame #1 {
            w520 = T18 {"error"=FALSE, "code"=0, "source"=""}  # No error
            n325 = property on="MG Enabled?" class="Bool (strict)"() -> ("Value"=w519:bool)  [unwired: 2 in, 2 out]
            n326 = case shown="True" w519 {
              tunnel: [w523 w540] -> w516
              tunnel: [w521 w524] -> w517
              tunnel: w520 -> [w523 w530]
              tunnel: [FALSE TRUE] -> _
              tunnel: w518 -> [w521 w535]
              frame False {
                # "MaxiGauge not connected"
              }
              frame True {
                n327 = call "Stop Display Busy AE.vi"("Action"=enum16{"Write", "Read"}."Write", "Error In"=w530, "Stop?"=FALSE) -> ("Error Out"=w525:errorcluster)  [unwired: 7 in, 1 out]
                n328 = call "MG- Scan ports.vi"("Error in"=w525, "RS232 port"=w535) -> ("Error out"=w527:errorcluster, "ID string"=→"Maxigauge ID":string, "VISA Refnum out"=w534:refnum<visa-resource-name>)  [unwired: 6 in, 1 out]
                n329 = call "Stop Display Busy AE.vi"("Action"=enum16{"Write", "Read"}."Write", "Error In"=w527, "Stop?"=TRUE) -> ()  [unwired: 7 in, 2 out]
                n330 = call "Display Busy.vi"("error in (no error)"=w525, "Title"="Trying to connect to the MaxiGauge") -> ()  [unwired: 8 in, 2 out]
                n331 = call "MG Get Channels Labels.vi"("MaxiGauge port"=w534) -> ("Array"=w538:string[], "MaxiGauge port"=w524:refnum<visa-resource-name>, "error out"=w540:errorcluster)  [unwired: 1 in]
                "MG port" <- w524
                n332 = Array To Cluster(array=w538) -> (cluster=→"Cluster":T33)
                n333 = for {
                  tunnel: w538 -> [w542] mode=indexing
                  i -> [w543]
                  n334 = property on="MaxiGauge" class="XYGraph (strict)"("Active Plot"=w543, "Plot.Plot Name"=w542) -> ()  [unwired: 2 in, 2 out]
                }
                n335 = Search 1D Array(1D array=w538, element="STIL") -> (index of element=w536:i32)  [unwired: 1 in]
                n336 = property on="MG  channel P8" class="Ring (strict)"("Value"=w536) -> ()  [unwired: 2 in, 2 out]
                n337 = property on="MG port number" class="VISAName"("Value"=w524) -> ()  [unwired: 2 in, 2 out]
              }
            }
            "MG error" <- w516
          }
          frame #2 {
            n338 = property on="PT1 port \nnumber" class="VISAName"() -> ("Value"=w547:refnum<visa-resource-name>)  [unwired: 2 in, 2 out]
            n339 = property on="PT1 Enabled?" class="Bool (strict)"() -> ("Value"=w553:bool)  [unwired: 2 in, 2 out]
            n340 = case shown="True" w553 {
              tunnel: w547 -> [_ w585]
              tunnel: [u16 0 ("Port Number out") w584] -> w544
              tunnel: [errorcluster {"status"=FALSE, "code"=0, "source"=""} ("Error out") w576] -> w552
              tunnel: [refnum<visa-resource-name> refnum ("VISA Refnum out") w573] -> w545
              frame False {
              }
              frame True {
                n341 = call "Stop Display Busy AE.vi"("Action"=enum16{"Write", "Read"}."Write", "Stop?"=FALSE) -> ("Error Out"=w574:errorcluster)  [unwired: 8 in, 1 out]
                n342 = property on="PT1 Bauds" class="DigNum (strict)"() -> ("Value"=w583:u32)  [unwired: 2 in, 2 out]
                n343 = property on="PT1 Address" class="DigNum (strict)"() -> ("Value"=w582:u8)  [unwired: 2 in, 2 out]
                n344 = call "PT-Scan ports.vi"("Error in"=w574, "PT Address"=w582, "Baud rate"=w583, "RS232 port"=w585) -> ("Error out"=w577:errorcluster, "Port Number out"=w584:u16, "serial Port out"=w573:refnum<visa-resource-name>)  [unwired: 3 in, 2 out]
                n345 = call "Display Busy.vi"("error in (no error)"=w574, "Title"="Trying to connect to PulseTube1") -> ()  [unwired: 8 in, 2 out]
                n346 = property on="PT1 port \nnumber" class="VISAName"("Value"=w573) -> ()  [unwired: 2 in, 2 out]
                n347 = call "Stop Display Busy AE.vi"("Action"=enum16{"Write", "Read"}."Write", "Error In"=w577, "Stop?"=TRUE) -> ("Error Out"=w576:errorcluster)  [unwired: 7 in, 1 out]
              }
            }
            "PT1 error" <- w552
            "PT1 port" <- w544
            n348 = property on="PT2 port \nnumber" class="VISAName"() -> ("Value"=w546:refnum<visa-resource-name>)  [unwired: 2 in, 2 out]
            n349 = property on="PT2 Enabled?" class="Bool (strict)"() -> ("Value"=w550:bool)  [unwired: 2 in, 2 out]
            n350 = Build Array(w545) -> (w551:refnum<visa-resource-name>[])
            n351 = case shown="True" w550 {
              tunnel: w546 -> [_ w569]
              tunnel: [u16 0 ("Port Number out") w568] -> w548
              tunnel: [errorcluster {"status"=FALSE, "code"=0, "source"=""} ("Error out") w557] -> w549
              tunnel: w551 -> [_ w565]
              frame False {
              }
              frame True {
                n352 = call "Stop Display Busy AE.vi"("Action"=enum16{"Write", "Read"}."Write", "Stop?"=FALSE) -> ("Error Out"=w561:errorcluster)  [unwired: 8 in, 1 out]
                n353 = property on="PT2 Bauds" class="DigNum (strict)"() -> ("Value"=w567:u32)  [unwired: 2 in, 2 out]
                n354 = property on="PT2 Address" class="DigNum (strict)"() -> ("Value"=w566:u8)  [unwired: 2 in, 2 out]
                n355 = call "PT-Scan ports.vi"("RS232 ports to skip"=w565, "Error in"=w561, "PT Address"=w566, "Baud rate"=w567, "RS232 port"=w569) -> ("Error out"=w558:errorcluster, "Port Number out"=w568:u16, "serial Port out"=w556:refnum<visa-resource-name>)  [unwired: 2 in, 2 out]
                n356 = call "Display Busy.vi"("error in (no error)"=w561, "Title"="Trying to connect to PulseTube2") -> ()  [unwired: 8 in, 2 out]
                n357 = property on="PT2 port \nnumber" class="VISAName"("Value"=w556) -> ()  [unwired: 2 in, 2 out]
                n358 = call "Stop Display Busy AE.vi"("Action"=enum16{"Write", "Read"}."Write", "Error In"=w558, "Stop?"=TRUE) -> ("Error Out"=w557:errorcluster)  [unwired: 7 in, 1 out]
              }
            }
            "PT2 error" <- w549
            "PT2 port" <- w548
          }
          frame #3 {
            n359 = disable-structure shown="Disabled" {
              disable-tunnel: w589 -> [w595 w603]
              disable-tunnel: w588 -> [w594 w602]
              disable-tunnel: [w593 w602] -> w587
              disable-tunnel: [w590 w603] -> w586
              frame Disabled {
                n360 = property on="S2 Enabled?" class="Bool (strict)"() -> ("Value"=w591:bool)  [unwired: 2 in, 2 out]
                n361 = property on="S1 Enabled?" class="Bool (strict)"() -> ("Value"=w592:bool)  [unwired: 2 in, 2 out]
                n362 = case shown="False" w592 {
                  tunnel: w595 -> [w599 w601]
                  tunnel: [w599 w600] -> w590
                  frame False {
                  }
                  frame True {
                    n363 = call "PV Initialize.vi"("VISA session in"=w601) -> ("VISA session out"=w600:refnum<visa-resource-name>)  [unwired: 9 in, 1 out]
                  }
                }
                n364 = case shown="False" w591 {
                  tunnel: w594 -> [w596 w598]
                  tunnel: [w596 w597] -> w593
                  frame False {
                  }
                  frame True {
                    n365 = call "PV Initialize.vi"("VISA session in"=w598) -> ("VISA session out"=w597:refnum<visa-resource-name>)  [unwired: 9 in, 1 out]
                  }
                }
              }
              frame Enabled {
              }
            }
          }
          frame #4 {
            w605 = T28."Page Enabled" ("Page Enabled State")
            w610 = u8 0 ("Disabled")
            w613 = u8 0 ("Disabled")
            n366 = property on="Configuration" class="Clust (strict)"("Disabled"=u8 2) -> ()  [unwired: 2 in, 2 out]
            n367 = property on="Buttons" class="Clust"("Disabled"=w613) -> ()  [unwired: 2 in, 2 out]
            n368 = property on="Buttons 2" class="Clust"("Disabled"=w613) -> ()  [unwired: 2 in, 2 out]
            n369 = local write "Start"(FALSE ("Start")) -> ()
            n370 = property on="Main Panel" class="TabCtl (strict)"("Disabled"=w610) -> ()  [unwired: 2 in, 2 out]
            n371 = property on="Main Panel" class="TabCtl (strict)"("Disabled"=w610) -> ()  [unwired: 2 in, 2 out]
            n372 = property on="Stop" class="Bool (strict)"("Disabled"=w610) -> ()  [unwired: 2 in, 2 out]
            n373 = property on="Error panel" class="TabCtl (strict)"("Disabled"=w610) -> ()  [unwired: 2 in, 2 out]
            n374 = property on="Side Panel" class="TabCtl (strict)"("Value"=enum32{"Main", "Settings", "Advanced"}."Main" ("Side Panel")) -> ("Pages"=w607:refnum<vi>[])  [unwired: 2 in, 2 out]
            n375 = Index Array(array=w607) -> (element #1=w608:refnum<vi>, element #2=w604:refnum<vi>, element #3=w609:refnum<vi>)  [unwired: 3 in]
            n376 = property class="Page"(reference=w608, "PageEnb"=w605) -> ()  [unwired: 1 in, 2 out]
            n377 = property class="Page"(reference=w604, "PageEnb"=w605) -> ()  [unwired: 1 in, 2 out]
            n378 = property class="Page"(reference=w609, "PageEnb"=w605) -> ()  [unwired: 1 in, 2 out]
          }
          frame #5 {
            n379 = Set Occurrence(w616) -> ()
            n380 = property on="Start" class="Bool (strict)"("Visible"=TRUE, "Disabled"=u8 2) -> ()  [unwired: 2 in, 2 out]
          }
        }
      }
      event "Stop": Value Change {
        w617 = u16 0 ("Port Number out")
        w618 = refnum<visa-resource-name> refnum ("PT port")
        n381 = event-data() -> ()  [unwired: 1 in, 6 out]
        n382 = call "Stop Display Busy AE.vi"("Action"=enum16{"Write", "Read"}."Write", "Stop?"=FALSE) -> ("Error Out"=w621:errorcluster)  [unwired: 8 in, 1 out]
        n383 = call "Display Busy.vi"("error in (no error)"=w621, "Title"="Stopping...") -> ()  [unwired: 8 in, 2 out]
        n384 = flat-sequence {
          tunnel: w628 -> [w635]
          tunnel: [w634] -> w623
          tunnel: w621 -> [w634]
          tunnel: w632 -> [w639]
          tunnel: w631 -> [w637]
          tunnel: w630 -> [w638]
          tunnel: w629 -> [w640]
          tunnel: [w636] -> w624
          tunnel: w623 -> [w636]
          tunnel: [w643] -> w625
          tunnel: w624 -> [w643]
          tunnel: w625 -> [w650]
          tunnel: [w649] -> w620
          tunnel: w620 -> [w655]
          tunnel: [w655] -> w619
          tunnel: w619 -> [_]
          frame #0 {
            n385 = Wait on Occurrence(2:w635) -> ()  [unwired: 2 in, 1 out]
          }
          frame #1 {
            n386 = VISA Close(VISA resource name=w639) -> ()  [unwired: 1 in, 1 out]
            n387 = VISA Close(VISA resource name=w637) -> ()  [unwired: 1 in, 1 out]
            n388 = VISA Close(VISA resource name=w638) -> ()  [unwired: 1 in, 1 out]
            n389 = VISA Close(VISA resource name=w640) -> ()  [unwired: 1 in, 1 out]
          }
          frame #2 {
            n390 = control-ref of="Configuration"() -> (w646:refnum<vi>)
            n391 = control-ref of="ADC scaling"() -> (w644:refnum<vi>)
            n392 = control-ref of="Log Options"() -> (w642:refnum<vi>)
            n393 = property on="Start" class="Bool (strict)"("Visible"=TRUE) -> ()  [unwired: 2 in, 2 out]
            n394 = Build Array(w646, w644, w642) -> (w647:refnum<vi>[])
            n395 = call "Save Load Settings to File by Ref with path.vi"("Array of Cluster References"=w647, "Action"=enum8{"Load", "Save"}."Save", "Configuration file"=path "C:/LC Data/Configuration/FP/FP config.ini" ("Relative path (.)")) -> ()  [unwired: 6 in, 1 out]
          }
          frame #3 {
            n396 = call "Stop Display Busy AE.vi"("Action"=enum16{"Write", "Read"}."Write", "Error In"=w650, "Stop?"=TRUE) -> ("Error Out"=w649:errorcluster)  [unwired: 7 in, 1 out]
            n397 = property on="Stop" class="Bool (strict)"("Value"=FALSE ("stop")) -> ()  [unwired: 2 in, 2 out]
          }
          frame #4 {
            n398 = Wait (ms)(milliseconds to wait=u32 500) -> ()  [unwired: 1 out]
          }
          frame #5 {
            n399 = Stop(stop? (T)=TRUE) -> ()
          }
        }
      }
      event "PT Start": Value Change {
        w665 = u16 54529 items=["Compressor START"=54529, "Compressor STOP"=50584, "Error Code"=26020, "Reset Max/Min"=54235] ("Command")
        n400 = event-data() -> ()  [unwired: 1 in, 6 out]
        n401 = property on="PT1 Address" class="DigNum (strict)"() -> ("Value"=w658:u8)  [unwired: 2 in, 2 out]
        n402 = property on="PT1 Bauds" class="DigNum (strict)"() -> ("Value"=w657:u32)  [unwired: 2 in, 2 out]
        n403 = call "PT Send Command.vi"("PT1 port"=w662, "PT Address"=w658, "PT Bauds"=w657, "Command"=w665) -> ()  [unwired: 1 in, 2 out]
      }
      event "PT Start 2": Value Change {
        w674 = u16 54529 items=["Compressor START"=54529, "Compressor STOP"=50584, "Error Code"=26020, "Reset Max/Min"=54235] ("Command")
        n404 = event-data() -> ()  [unwired: 1 in, 6 out]
        n405 = property on="PT2 Address" class="DigNum (strict)"() -> ("Value"=w667:u8)  [unwired: 2 in, 2 out]
        n406 = property on="PT2 Bauds" class="DigNum (strict)"() -> ("Value"=w666:u32)  [unwired: 2 in, 2 out]
        n407 = call "PT Send Command.vi"("PT1 port"=w668, "PT Address"=w667, "PT Bauds"=w666, "Command"=w674) -> ()  [unwired: 1 in, 2 out]
      }
      event "PT_stop": Value Change {
        w683 = u16 50584 items=["Compressor START"=54529, "Compressor STOP"=50584, "Error Code"=26020, "Reset Max/Min"=54235] ("Command")
        n408 = event-data() -> ()  [unwired: 1 in, 1 out]
        n409 = property on="PT1 Address" class="DigNum (strict)"() -> ("Value"=w676:u8)  [unwired: 2 in, 2 out]
        n410 = property on="PT1 Bauds" class="DigNum (strict)"() -> ("Value"=w675:u32)  [unwired: 2 in, 2 out]
        n411 = call "PT Send Command.vi"("PT1 port"=w680, "PT Address"=w676, "PT Bauds"=w675, "Command"=w683) -> ()  [unwired: 1 in, 2 out]
      }
      event "PT_stop 2": Value Change {
        w692 = u16 50584 items=["Compressor START"=54529, "Compressor STOP"=50584, "Error Code"=26020, "Reset Max/Min"=54235] ("Command")
        n412 = event-data() -> ()  [unwired: 1 in, 1 out]
        n413 = property on="PT2 Address" class="DigNum (strict)"() -> ("Value"=w685:u8)  [unwired: 2 in, 2 out]
        n414 = property on="PT2 Bauds" class="DigNum (strict)"() -> ("Value"=w684:u32)  [unwired: 2 in, 2 out]
        n415 = call "PT Send Command.vi"("PT1 port"=w686, "PT Address"=w685, "PT Bauds"=w684, "Command"=w692) -> ()  [unwired: 1 in, 2 out]
      }
      event "PT Error Code": Value Change {
        n416 = event-data() -> ("OldVal"=w701:i32, "NewVal"=w697:i32)  [unwired: 1 in]
        n417 = Not Equal?(x=w701, y=w697) -> (x != y?=w700:bool)
        n418 = global read "ErrCodeStatusLkup.vi" "Error code/name/description Firmware V1.5"() -> (w698:string)
        n419 = case shown="Default" w697 {
          tunnel: w699 -> [_ w712]
          frame 0, 14..23 {
            # "No Error or Warning"
            "Attempts Counter" <- u16 0 ("Attempts Counter")
          }
          frame Default {
            # "Error"
            n420 = local read "Attempts Counter"() -> (w718:u16)
            n421 = Less?(x=w718, y="Attempts") -> (x < y?=w715:bool)
            n422 = And(x=w715, y="Restart PT on Error?") -> (x .and. y?=w714:bool)
            n423 = case shown="True" w714 {
              tunnel: "Time delay" -> [_ w720]
              tunnel: w712 -> [_ w719]
              frame False {
              }
              frame True {
                n424 = flat-sequence {
                  tunnel: w719 -> [w721]
                  tunnel: w720 -> [w725]
                  frame #0 {
                    n425 = call "PT start.vi"("PT1 port"=w721) -> ()  [unwired: 1 in, 2 out]
                  }
                  frame #1 {
                    n426 = local read "Attempts Counter"() -> (w723:u16)
                    n427 = Increment(x=w723) -> (x+1=w722:u16)
                    n428 = local write "Attempts Counter"(w722) -> ()
                  }
                  frame #2 {
                    n429 = Multiply(x=w725, y=u16 1000) -> (x*y=w726:u16)
                    n430 = Wait (ms)(milliseconds to wait=w726) -> ()  [unwired: 1 out]
                  }
                }
              }
            }
          }
        }
        n431 = Pick Line(multi-line string=w698, line index=w697) -> (output string=w696:string)  [unwired: 1 in]
        "PT Error" <- w696
        n432 = case shown="True" w700 {
          tunnel: w697 -> [_ w707]
          tunnel: w696 -> [_ w704]
          frame False {
          }
          frame True {
            n433 = Format Date/Time String() -> (date/time string=w705:string)  [unwired: 3 in]
            n434 = Number To Decimal String(number=w707) -> (decimal integer string=w706:string)  [unwired: 1 in]
            n435 = Build Array(w705, w706, w704) -> (w708:string[])
            n436 = feedback #1() -> (w709:string[][])  [unwired: 1 in]
            "Error Log" <- w709
            n437 = Build Array (concatenate)(w709, w708) -> (w710:string[][])
            n438 = feedback-in #1(w710) -> ()
          }
        }
      }
      event "PT_ResetValues": Value Change {
        w735 = u16 54235 items=["Compressor START"=54529, "Compressor STOP"=50584, "Error Code"=26020, "Reset Max/Min"=54235] ("Command")
        n439 = event-data() -> ()  [unwired: 1 in, 1 out]
        n440 = property on="PT1 Address" class="DigNum (strict)"() -> ("Value"=w728:u8)  [unwired: 2 in, 2 out]
        n441 = property on="PT1 Bauds" class="DigNum (strict)"() -> ("Value"=w727:u32)  [unwired: 2 in, 2 out]
        n442 = call "PT Send Command.vi"("PT1 port"=w732, "PT Address"=w728, "PT Bauds"=w727, "Command"=w735) -> ()  [unwired: 1 in, 2 out]
      }
      event "PT_ResetValues 2": Value Change {
        w744 = u16 54235 items=["Compressor START"=54529, "Compressor STOP"=50584, "Error Code"=26020, "Reset Max/Min"=54235] ("Command")
        n443 = event-data() -> ()  [unwired: 1 in, 1 out]
        n444 = property on="PT2 Address" class="DigNum (strict)"() -> ("Value"=w737:u8)  [unwired: 2 in, 2 out]
        n445 = property on="PT2 Bauds" class="DigNum (strict)"() -> ("Value"=w736:u32)  [unwired: 2 in, 2 out]
        n446 = call "PT Send Command.vi"("PT1 port"=w738, "PT Address"=w737, "PT Bauds"=w736, "Command"=w744) -> ()  [unwired: 1 in, 2 out]
      }
      event "Buttons": Value Change {
        n447 = event-data() -> ("NewVal"=w753:T3)  [unwired: 1 in, 5 out]
        n448 = Cluster To Array(cluster=w753) -> (array=w752:bool[])
        n449 = while {
          tunnel: w752 -> [w757] mode=indexing
          tunnel: [w756] -> w751
          i -> [w756]
          stop <- w757 stop-if-true
        }
        n450 = Increment(x=w751) -> (x+1=w750:i32)
        n451 = call "BP togglekey.vi"("keynumber"=w750, "FrontPanel port"=w749) -> ("FrontPanel port"=w748:refnum<visa-resource-name>)  [unwired: 2 in, 1 out]
      }
      event "Buttons 2": Value Change {
        n452 = event-data() -> ("NewVal"=w766:T3)  [unwired: 1 in, 5 out]
        n453 = Cluster To Array(cluster=w766) -> (array=w765:bool[])
        n454 = while {
          tunnel: w765 -> [w770] mode=indexing
          tunnel: [w769] -> w764
          i -> [w769]
          stop <- w770 stop-if-true
        }
        n455 = Increment(x=w764) -> (x+1=w763:i32)
        n456 = call "BP togglekey.vi"("keynumber"=w763, "FrontPanel port"=w762) -> ("FrontPanel port"=w761:refnum<visa-resource-name>)  [unwired: 2 in, 1 out]
      }
      event "Button": Value Change {
        n457 = event-data() -> ()  [unwired: 1 in, 6 out]
        n458 = call "BP togglekey.vi"("keynumber"="Button", "FrontPanel port"=w776) -> ("FrontPanel port"=w775:refnum<visa-resource-name>)  [unwired: 2 in, 1 out]
      }
      event "SET VALUES": Value Change {
        n459 = event-data() -> ("OldVal"=w785:bool)  [unwired: 1 in, 5 out]
        n460 = property on="SET VALUES" class="Bool (strict)"("Value"=w785) -> ()  [unwired: 2 in, 2 out]
        n461 = stacked-sequence {
          tunnel: w780 -> [w791 w805 w820 w838 w853 w868]
          tunnel: [w787 _ _ _ _ _] -> w779
          frame #0 {
            n462 = local read "P6&7 Settings"() -> (w790:T13)
            n463 = local read "P6&7 limits"() -> (w789:T13)
            n464 = Not Equal?(x=w790, y=w789) -> (x != y?=w788:bool)
            n465 = case shown="True" w788 {
              tunnel: w791 -> [w793 w800]
              tunnel: [w793 w799] -> w787
              frame False {
                n466 = control-ref of="P6&7 Settings"() -> (w792:refnum<vi>)
                n467 = call "FP check parameters error.vi"("Clust Refnum"=w792) -> ()  [unwired: 6 in, 1 out]
              }
              frame True {
                n468 = control-ref of="P6&7 Settings"() -> (w796:refnum<vi>)
                n469 = call "BP Set Config.vi"("GHS Settings"="P6&7 Settings", "FrontPanel port"=w800) -> ("error out"=w798:T18, "FrontPanel port"=w804:refnum<visa-resource-name>)  [unwired: 2 in]
                n470 = call "FP check parameters error.vi"("error in"=w798, "Clust Refnum"=w796) -> ("error out"=w797:errorcluster)  [unwired: 5 in]
                n471 = call "BP query settings.vi"("error in"=w797, "FrontPanel port"=w804) -> ("error out"=w795:T18, "array of 4 x 16 bit unsigned"=w802:u16[], "BP response"=→"Panel response":string, "FrontPanel port"=w799:refnum<visa-resource-name>)  [unwired: 2 in]
                n472 = Array To Cluster(array=w802) -> (cluster=→"P6&7 limits":T30)
                n473 = local write "FP error"(w795) -> ()
              }
            }
          }
          frame #1 {
            n474 = local read "P5 Settings"() -> (w807:cluster{"P6 low":u16, "P6 high":u16})
            n475 = local read "P5 limits"() -> (w808:cluster{"P5 C1":u16, "P5 C2":u16})
            n476 = Not Equal?(x=w807, y=w808) -> (x != y?=w806:bool)
            n477 = case shown="True" w806 {
              tunnel: w805 -> [_ w815]
              frame False {
                n478 = control-ref of="P5 Settings"() -> (w809:refnum<vi>)
                n479 = call "FP check parameters error.vi"("Clust Refnum"=w809) -> ()  [unwired: 6 in, 1 out]
              }
              frame True {
                n480 = control-ref of="P5 Settings"() -> (w812:refnum<vi>)
                n481 = call "BP Set P5.vi"("P5 Settings"="P5 Settings", "FrontPanel port in"=w815) -> ("error out"=w819:errorcluster, "FrontPanel port out"=w818:refnum<visa-resource-name>)  [unwired: 2 in]
                n482 = call "FP check parameters error.vi"("error in"=w819, "Clust Refnum"=w812) -> ("error out"=w813:errorcluster)  [unwired: 5 in]
                n483 = call "BP query P5.vi"("error in"=w813, "FrontPanel port"=w818) -> ("error out"=w811:T18, "array of 2 x 16 bit unsigned"=w817:u16[], "BP response"=w810:string)  [unwired: 2 in, 1 out]
                n484 = Array To Cluster(array=w817) -> (cluster=→"P5 limits":T31)
                n485 = local write "Panel response"(w810) -> ()
                n486 = local write "FP error"(w811) -> ()
              }
            }
          }
          frame #2 {
            n487 = local read "NCP5 Settings"() -> (w822:T10)
            n488 = local read "NCP5 limits"() -> (w823:T12)
            n489 = Not Equal?(x=w822, y=w823) -> (x != y?=w821:bool)
            n490 = case shown="True" w821 {
              tunnel: w820 -> [_ w830]
              frame False {
                n491 = control-ref of="NCP5 Settings"() -> (w824:refnum<vi>)
                n492 = call "FP check parameters error.vi"("Clust Refnum"=w824) -> ()  [unwired: 6 in, 1 out]
              }
              frame True {
                n493 = control-ref of="NCP5 Settings"() -> (w827:refnum<vi>)
                n494 = call "BP Set NCP5.vi"("NCP5 Settings"="NCP5 Settings", "FrontPanel port in"=w830) -> ("error out"=w829:errorcluster, "FrontPanel port out"=w834:refnum<visa-resource-name>)  [unwired: 2 in]
                n495 = call "FP check parameters error.vi"("error in"=w829, "Clust Refnum"=w827) -> ("error out"=w828:errorcluster)  [unwired: 5 in]
                n496 = call "BP query NCP5.vi"("error in"=w828, "FrontPanel port"=w834) -> ("error out"=w826:T18, "array of 3 x 16 bit unsigned"=w832:u16[], "BP response"=w825:string)  [unwired: 2 in, 1 out]
                n497 = local write "Panel response"(w825) -> ()
                n498 = Array To Cluster(array=w832) -> (cluster=→"NCP5 limits":T32)
                n499 = local write "FP error"(w826) -> ()
              }
            }
          }
          frame #3 {
            n500 = local read "NCP5B Settings"() -> (w835:cluster{"P6 low":u16})
            n501 = local read "NCP5B limits"() -> (w836:cluster{"P5 NC4":u16})
            n502 = Not Equal?(x=w835, y=w836) -> (x != y?=w837:bool)
            n503 = case shown="True" w837 {
              tunnel: w838 -> [_ w845]
              frame False {
                n504 = control-ref of="NCP5B Settings"() -> (w839:refnum<vi>)
                n505 = call "FP check parameters error.vi"("Clust Refnum"=w839) -> ()  [unwired: 6 in, 1 out]
              }
              frame True {
                n506 = control-ref of="NCP5B Settings"() -> (w842:refnum<vi>)
                n507 = call "BP Set NCP5B.vi"("NCP5B"="NCP5B Settings", "FrontPanel port in"=w845) -> ("error out"=w844:errorcluster, "FrontPanel port out"=w846:refnum<visa-resource-name>)  [unwired: 2 in]
                n508 = call "FP check parameters error.vi"("error in"=w844, "Clust Refnum"=w842) -> ("error out"=w843:errorcluster)  [unwired: 5 in]
                n509 = call "BP query NCP5B.vi"("error in"=w843, "FrontPanel port"=w846) -> ("error out"=w841:T18, "array of 3 x 16 bit unsigned"=w847:u16[], "BP response"=w840:string)  [unwired: 2 in, 1 out]
                n510 = local write "Panel response"(w840) -> ()
                n511 = Array To Cluster(array=w847) -> (cluster=→"NCP5B limits":cluster{"array of 3 x 16 bit unsigned[0]":u16})
                n512 = local write "FP error"(w841) -> ()
              }
            }
          }
          frame #4 {
            n513 = local read "REC Settings"() -> (w851:T10)
            n514 = local read "REC limits"() -> (w852:T11)
            n515 = Not Equal?(x=w851, y=w852) -> (x != y?=w850:bool)
            n516 = case shown="True" w850 {
              tunnel: w853 -> [_ w860]
              frame False {
                n517 = control-ref of="REC Settings"() -> (w854:refnum<vi>)
                n518 = call "FP check parameters error.vi"("Clust Refnum"=w854) -> ()  [unwired: 6 in, 1 out]
              }
              frame True {
                n519 = control-ref of="REC Settings"() -> (w857:refnum<vi>)
                n520 = call "BP Set REC.vi"("NCP5 Settings"="REC Settings", "FrontPanel port in"=w860) -> ("error out"=w859:errorcluster, "FrontPanel port out"=w861:refnum<visa-resource-name>)  [unwired: 2 in]
                n521 = call "FP check parameters error.vi"("error in"=w859, "Clust Refnum"=w857) -> ("error out"=w858:errorcluster)  [unwired: 5 in]
                n522 = call "BP Query REC.vi"("error in"=w858, "FrontPanel port"=w861) -> ("error out"=w856:T18, "array of 3 x 16 bit unsigned"=w863:u16[], "BP response"=w855:string)  [unwired: 2 in, 1 out]
                n523 = local write "Panel response"(w855) -> ()
                n524 = Array To Cluster(array=w863) -> (cluster=→"REC limits":T32)
                n525 = local write "FP error"(w856) -> ()
              }
            }
          }
          frame #5 {
            n526 = local read "S1&2 Settings"() -> (w865:cluster{"Enum":enum16{"OFF", "ON"}})
            n527 = local read "S1&2 limits"() -> (w866:cluster{"S1&S2":enum16{"OFF", "ON"}})
            n528 = Not Equal?(x=w865, y=w866) -> (x != y?=w867:bool)
            n529 = case shown="True" w867 {
              tunnel: w868 -> [_ w877]
              frame False {
                n530 = control-ref of="S1&2 Settings"() -> (w869:refnum<vi>)
                n531 = call "FP check parameters error.vi"("Clust Refnum"=w869) -> ()  [unwired: 6 in, 1 out]
              }
              frame True {
                n532 = control-ref of="S1&2 Settings"() -> (w872:refnum<vi>)
                n533 = call "BP Set Turbo.vi"("S1&2 Settings"="S1&2 Settings", "FrontPanel port in"=w877) -> ("error out"=w874:errorcluster, "FrontPanel port out"=w878:refnum<visa-resource-name>)  [unwired: 2 in]
                n534 = call "FP check parameters error.vi"("error in"=w874, "Clust Refnum"=w872) -> ("error out"=w873:errorcluster)  [unwired: 5 in]
                n535 = call "BP Query Turbo.vi"("error in"=w873, "FrontPanel port"=w878) -> ("error out"=w871:T18, "array of 3 x 16 bit unsigned"=w879:u16[], "BP response"=w870:string)  [unwired: 2 in, 1 out]
                n536 = local write "Panel response"(w870) -> ()
                n537 = Array To Cluster(array=w879) -> (cluster=→"S1&2 limits":cluster{"array of 3 x 16 bit unsigned[0]":u16})
                n538 = local write "FP error"(w871) -> ()
              }
            }
          }
        }
      }
      event "Log Options.Plot data": Value Change {
        n539 = event-data() -> ("NewVal"=w886:bool)  [unwired: 1 in, 5 out]
        n540 = property on="Main Panel" class="TabCtl (strict)"() -> ("Pages"=w889:refnum<vi>[])  [unwired: 2 in, 2 out]
        n541 = Index Array(array=w889, index=2) -> (element=w887:refnum<vi>)
        n542 = property class="Page"(reference=w887, "PageVis"=w886) -> ()  [unwired: 1 in, 2 out]
      }
      event "Autoconf": Value Change {
        n543 = event-data() -> ()  [unwired: 1 in, 6 out]
      }
      event "Configuration": Value Change {
        n544 = event-data() -> ()  [unwired: 1 in, 6 out]
        n545 = VISA Close(VISA resource name=w907) -> ()  [unwired: 1 in, 1 out]
        n546 = VISA Close(VISA resource name=w908) -> ()  [unwired: 1 in, 1 out]
        n547 = VISA Close(VISA resource name=w905) -> ()  [unwired: 1 in, 1 out]
        n548 = VISA Close(VISA resource name=w903) -> ()  [unwired: 1 in, 1 out]
        n549 = Unbundle By Name("Configuration") -> ("PT1 port number"=w897:refnum<visa-resource-name>, "PT2 port number"=w899:refnum<visa-resource-name>, "FP port number"=w909:refnum<visa-resource-name>, "MG port number"=w906:refnum<visa-resource-name>, "S1 port"=w904:refnum<visa-resource-name>, "S2 port"=w902:refnum<visa-resource-name>)
        n550 = call "VISA to RS232 Port Nr.vi"("VISA Resource Name"=w897) -> ("Port Number"=w901:u8)  [unwired: 1 in]
        n551 = call "VISA to RS232 Port Nr.vi"("VISA Resource Name"=w899) -> ("Port Number"=w900:u8)  [unwired: 1 in]
        n552 = Increment(x=w901) -> (x+1=w896:u8)
        n553 = Increment(x=w900) -> (x+1=w898:u8)
      }
      event "Type": Value Change {
        n554 = event-data() -> ("NewVal"=w914:enum32{"Wet", "CF"})  [unwired: 1 in, 5 out]
        n555 = case shown="\"CF\", Default" w914 {
          tunnel: ["COMPRESSOR" ("Label.Text") "AUX 2" ("Label.Text")] -> w919
          tunnel: [TRUE ("Visible") FALSE ("Visible")] -> w915
          tunnel: ["From\nProbe" ("Text.Text") "From\nDewar" ("Text.Text")] -> w913
          tunnel: ["From\nOVC" ("Text.Text") "From\n1K pot" ("Text.Text")] -> w912
          frame "CF", Default {
          }
          frame "Wet" {
          }
        }
        n556 = property on="Main Panel" class="TabCtl (strict)"() -> ("Pages"=w918:refnum<vi>[])  [unwired: 2 in, 2 out]
        n557 = Index Array(array=w918, index=1) -> (element=w916:refnum<vi>)
        n558 = property on="COMPR/AUX 2" class="Bool (strict)"("Caption.Text"=w919) -> ()  [unwired: 2 in, 2 out]
        n559 = property on="String 3" class="Str"("Text.Text"=w913) -> ()  [unwired: 2 in, 2 out]
        n560 = property on="String" class="Str"("Text.Text"=w912) -> ()  [unwired: 2 in, 2 out]
        n561 = property on="BYPASS" class="Bool (strict)"("Visible"=w915) -> ()  [unwired: 2 in, 2 out]
        n562 = property on="PT STATUS" class="Bool (strict)"("Visible"=w915) -> ()  [unwired: 2 in, 2 out]
        n563 = property class="Page"(reference=w916, "PageVis"=w915) -> ()  [unwired: 1 in, 2 out]
        n564 = property on="String 4" class="Str"("Text.Text"=w913) -> ()  [unwired: 2 in, 2 out]
        n565 = property on="String 2" class="Str"("Text.Text"=w912) -> ()  [unwired: 2 in, 2 out]
      }
      event "Panel Layout": Value Change {
        n566 = event-data() -> ("NewVal"=w939:enum32{"OLD", "NEW"})  [unwired: 1 in, 5 out]
        n567 = property on="FP type" class="TabCtl (strict)"("Value"=w939) -> ()  [unwired: 2 in, 2 out]
      }
      event "FP Status bits": Value Change {
        n568 = event-data() -> ("OldVal"=w948:u32[], "NewVal"=w947:u32[])  [unwired: 1 in, 4 out]
        n569 = Not Equal?(x=w948, y=w947) -> (x != y?=w946:bool)
        n570 = case shown="True" w946 {
          frame False {
          }
          frame True {
            "ForceSave" <- TRUE ("ForceSave")
          }
        }
      }
      event "Front Panel", "MaxiGauge": Shortcut Menu Activation? {
        w954 = string[] ["Log Y"] ("item names")
        w966 = string[] ["Autoscale XY"] ("item names")
        n571 = event-data() -> ("MenuRef"=w952:refnum<k9>, "CtlRef"=w951:refnum<vi>)  [unwired: 1 in]
        n572 = Insert Menu Items(4:10, 7:w966, 8:w966, 9:w952) -> (3:w953:refnum<k9>)  [unwired: 2 in, 2 out]
        n573 = property class="XYGraph (strict)"(reference=w951) -> ("YScale.Mapping Mode"=w957:u8)  [unwired: 1 in, 2 out]
        n574 = Insert Menu Items(4:13, 7:w954, 8:w954, 9:w953) -> (3:w956:refnum<k9>)  [unwired: 2 in, 2 out]
        n575 = Not Equal To 0?(x=w957) -> (x != 0?=w958:bool)
        n576 = Set Menu Item Info(6:w958, 7:"Log Y", 11:w956) -> ()  [unwired: 4 in, 2 out]
        n577 = event-data() -> ()  [unwired: 2 in, 1 out]
      }
      event "Front Panel", "MaxiGauge": Shortcut Menu Selection (User) {
        n578 = event-data() -> ("CtlRef"=w970:refnum<vi>, "ItemTag"=w976:string)  [unwired: 1 in]
        n579 = Type Cast(type=refnum<vi> refnum ("R-Plot 0"), x=w970) -> (*(type *) &x=w969:refnum<vi>)
        n580 = case shown="\"Log Y\"" w976 {
          tunnel: w969 -> [_ w977 w979]
          frame Default {
          }
          frame "Autoscale XY" {
            w978 = u8 2 ("X Scale.Scale Fit")
            n581 = property class="XYGraph (strict)"(reference=w977, "XScale.ScaleFit"=w978, "YScale.ScaleFit"=w978) -> ()  [unwired: 1 in, 2 out]
          }
          frame "Log Y" {
            n582 = property class="XYGraph (strict)"(reference=w979) -> (reference out=w980:refnum<vi>, "YScale.Mapping Mode"=w981:u8)  [unwired: 1 in, 1 out]
            n583 = Equal To 0?(x=w981) -> (x = 0?=w982:bool)
            n584 = Boolean To (0,1)(Boolean=w982) -> (0, 1=w983:i16)
            n585 = property class="XYGraph (strict)"(reference=w980, "YScale.Mapping Mode"=w983) -> ()  [unwired: 1 in, 2 out]
          }
        }
      }
      event "Front Panel", "MaxiGauge": Scale Range Change {
        w991 = u8 0 ("X Scale.Scale Fit")
        n586 = event-data() -> ("CtlRef"=w990:refnum<vi>)  [unwired: 1 in, 7 out]
        n587 = property class="XYGraph (strict)"(reference=w990, "XScale.ScaleFit"=w991, "YScale.ScaleFit"=w991) -> ()  [unwired: 1 in, 2 out]
      }
      event "Reset Error": Value Change {
        n588 = event-data() -> ()  [unwired: 1 in, 6 out]
        n589 = property on="Device address S1" class="DigNum (strict)"() -> ("Value"=w994:u8)  [unwired: 2 in, 2 out]
        n590 = call "PV Error Reset.vi"("Adress of unit"=w994, "VISA session"=w999) -> ("VISA resource out"=w993:refnum<visa-resource-name>)  [unwired: 8 in, 1 out]
      }
      event "Reset Error 2": Value Change {
        n591 = event-data() -> ()  [unwired: 1 in, 6 out]
        n592 = property on="Device address S2" class="DigNum (strict)"() -> ("Value"=w1002:u8)  [unwired: 2 in, 2 out]
        n593 = call "PV Error Reset.vi"("Adress of unit"=w1002, "VISA session"=w1007) -> ("VISA resource out"=w1001:refnum<visa-resource-name>)  [unwired: 8 in, 1 out]
      }
      event "Configuration.S1 Enabled?": Value Change {
        n594 = event-data() -> ("NewVal"=w1018:bool)  [unwired: 1 in, 5 out]
        n595 = Not(x=w1018) -> (.not. x?=w1017:bool)
        n596 = Boolean To (0,1)(Boolean=w1017) -> (0, 1=w1016:i16)
        n597 = Multiply(x=i16 2, y=w1016) -> (x*y=w1014:i16)
        n598 = property on="S1" class="TabCtl (strict)"("Disabled"=w1014) -> ()  [unwired: 2 in, 2 out]
      }
      event "Configuration.S2 Enabled?": Value Change {
        n599 = event-data() -> ("NewVal"=w1026:bool)  [unwired: 1 in, 5 out]
        n600 = Not(x=w1026) -> (.not. x?=w1029:bool)
        n601 = Boolean To (0,1)(Boolean=w1029) -> (0, 1=w1028:i16)
        n602 = Multiply(x=i16 2, y=w1028) -> (x*y=w1025:i16)
        n603 = property on="S2" class="TabCtl (strict)"("Disabled"=w1025) -> ()  [unwired: 2 in, 2 out]
      }
      event "Configuration.PT1 Enabled?", "Configuration.PT2 Enabled?": Value Change {
        n604 = event-data() -> ()  [unwired: 1 in, 6 out]
        n605 = property on="PT1 Enabled?" class="Bool (strict)"() -> ("Value"=w1031:bool)  [unwired: 2 in, 2 out]
        n606 = property on="PT2 Enabled?" class="Bool (strict)"() -> ("Value"=w1030:bool)  [unwired: 2 in, 2 out]
        n607 = property on="Main Panel" class="TabCtl (strict)"() -> ("Pages"=w1034:refnum<vi>[])  [unwired: 2 in, 2 out]
        n608 = Or(x=w1031, y=w1030) -> (x .or. y?=w1032:bool)
        n609 = Index Array(array=w1034) -> (element #2=w1033:refnum<vi>)  [unwired: 2 in, 1 out]
        n610 = property class="Page"(reference=w1033, "PageVis"=w1032) -> ()  [unwired: 1 in, 2 out]
      }
      event "Boolean 2": Value Change {
        n611 = event-data() -> ("NewVal"=w1047:bool)  [unwired: 1 in, 5 out]
        n612 = case shown="False" w1047 {
          frame True {
            n613 = property class="VI"() -> ("Front Panel.PanelBounds"=w1048:T34)  [unwired: 2 in, 2 out]
            n614 = Unbundle By Name(w1048) -> ("Left"=w1054:i16, "Top"=w1051:i16)
            n615 = Add(x=i16 955 ("right"), y=w1054) -> (x+y=w1053:i16)
            n616 = Add(x=w1051, y=i16 730) -> (x+y=w1049:i16)
            n617 = Bundle By Name(cluster=w1048, "Right"=w1053, "Bottom"=w1049) -> (w1055:T34)
            n618 = property class="VI"("Front Panel.PanelBounds"=w1055) -> ()  [unwired: 2 in, 2 out]
          }
          frame False {
            n619 = property class="VI"() -> ("Front Panel.PanelBounds"=w1056:T34)  [unwired: 2 in, 2 out]
            n620 = Unbundle By Name(w1056) -> ("Left"=w1062:i16, "Top"=w1059:i16)
            n621 = Add(x=i16 1259 ("right"), y=w1062) -> (x+y=w1061:i16)
            n622 = Add(x=w1059, y=i16 730) -> (x+y=w1057:i16)
            n623 = Bundle By Name(cluster=w1056, "Right"=w1061, "Bottom"=w1057) -> (w1063:T34)
            n624 = property class="VI"("Front Panel.PanelBounds"=w1063) -> ()  [unwired: 2 in, 2 out]
          }
        }
      }
      event "FP Plots Select", "MG Plots Select": Value Change {
        n625 = event-data() -> ()  [unwired: 1 in, 6 out]
        n626 = local write "ForceSave"(TRUE ("ForceSave")) -> ()
      }
      event "SendCMD": Value Change {
        n627 = event-data() -> ()  [unwired: 1 in, 6 out]
        n628 = call "BP Send Command.vi"("String"="Command", "FrontPanel port in"=w1074) -> ("string after ack"=→"Response":string, "FrontPanel port out"=w1073:refnum<visa-resource-name>)  [unwired: 1 in, 1 out]
      }
    }
  }
